vi "eyecat MAX v2_JS-Demo.vi"() -> ()   [LabVIEW 2014]
doc: "This VI is an upgrade from the WIN 1_v4 that implements the ageing subrutine"
uses:
  Buttons/String output.ctl
  <vilib>/Utility/miscctls.llb/LVRowAndColumnTypeDef.ctl
  Buttons/Numeric control.ctl
  Buttons/String input.ctl
  Buttons/Numeric indicator.ctl
  Controls Win/Control 3.ctl
  <vilib>/Platform/TimedLoop/XDataNode/nitl_modes.ctl
  <vilib>/Platform/TimedLoop/XDataNode/timing_clust.ctl
  <vilib>/Platform/TimedLoop/XDataNode/wakeup.ctl
  <vilib>/Utility/file.llb/Read From Spreadsheet File (DBL).vi
  <vilib>/Utility/file.llb/Write To Spreadsheet File (string).vi
  <vilib>/Utility/file.llb/Read From Spreadsheet File (string).vi
  <vilib>/regexp/Match Regular Expression.xnode
  <vilib>/Platform/TimedLoop/XDataNode/XDataNode.xnode
  <vilib>/Platform/TimedLoop/XDataNode/XDNodeRunTimeDep.lvlib
panel:
  in  "System Guide":bool
  in  "Mean(Off)/Interval(On) 5":bool
  in  "System Band":dbl=1.04
  in  "System Sync":i32
  in  "Heat Guide":bool
  in  "Mean(Off)/Interval(On) 4":bool
  in  "Heat Band %":dbl=1.04
  in  "Heat Sync":i32
  in  "Lambda Guide":bool
  in  "Mean(Off)/Interval(On) 3":bool
  in  "Lambda Band %":dbl=1.04
  in  "Lambda Sync":i32
  in  "FlowGuide":bool
  in  "Mean(Off)/Interval(On) 2":bool
  in  "Flow Band %":dbl=1.04
  in  "Flow Sync":i32
  in  "Execute Leak Test Button":bool
  in  "Stop Test Button":bool
  in  "Start Test Button":bool
  in  "Log Test Button":bool
  in  "Boolean":bool
  in  "MKS":bool
  in  "7170":bool
  out "Emissions":dbl[](array[numeric])
  in  "Temperature Sync":i32
  in  "TempGuide":bool
  in  "Temp Band %":dbl=1.04
  in  "Mean(Off)/Interval(On)":bool
  in  "MKS":bool
  out "output cluster":T2
  out "Lambda":dbl[](array[numeric])
  out "MKS HC":dbl
  in  "HC Index":i32
  in  "MFC Number":i32
  out "Open/Closed \nLoop":dbl[](array[numeric])
  out "Air Cyc 2":dbl[](array[numeric])
  in  "Cycle size":i32
  out "MFC Setpoint/Delivery":dynamicdata(graph)
  out "ExtAnDn":bool
  out "ExtAnUp":bool
  out "HC Cyc 2":dbl[](array[numeric])
  out "SO Valve 2":dbl[](array[numeric])
  out "SO Valve 1":dbl[](array[numeric])
  out "Air Bal":dbl[](array[numeric])
  out "HC Bal":dbl[](array[numeric])
  out "Air Cyc 1":dbl[](array[numeric])
  out "HC Cyc 1":dbl[](array[numeric])
  out "File name":string
  out "Log?":bool
  out "Advanced Logging":bool
  out "Connected":bool
  out "MKS 1":i16
  out "MKS 2":i16
  out "Furnace temp 2":dbl
  out "Full system?":bool
  out "Log interval (seconds)":T1
  in  "Flow rate Age":dbl
  in  "Inlet temp Age":dbl
  out "Stopped?":bool
  in  "Stop Cmd":T1
  out "Connected?":bool
  out "Error":dbl
  out "Iteration Duration":i64
  out "Finished Late? [i-1]":bool
  in  "SO2 ppm":dbl
  out "Furnace temp 1":dbl
  out "stop 2":bool
  in  "Enum 1":i16=1
  in  "Acknowledge":bool
  out "Test number":u16
  out "Flag1":bool=TRUE
  out "EditPos Subc":T3
  out "Flag 2":bool=TRUE
  in  "Tab Control":T4(tab)
  in  "Leak Test":bool
  in  "Stop Test":bool
  in  "Log Test Data":bool
  in  "Start":bool
  in  "Adv Settings":bool
  out "Doors Unlocked":bool
  in  "Temperature Limit (°C)":T1=800.0 min=0.0 max=1200.0 step=1.0
  in  "File Name":T5="Test"
  in  "File Path":path=path "C:/DATA LOG"
  out "Fail":bool
  out "Pass":bool
  in  "Select Test Type":T6(radio)
  out "Standby":bool
  out "Doors Open":bool
  out "Extractor Fan On":bool
  out "Test In Progress":bool
  out "Cool Down":bool
  out "System Alarm":bool
  in  "Inlet Temperature (°C)":T1=400.0 min=350.0 max=1000.0 step=1.0
  in  "Inlet LAMBDA Rich":T1=0.9 min=0.85 max=0.96 step=0.001
  in  "Inlet LAMBDA Lean":T1=1.2 min=1.02 max=3.0 step=0.001
  in  "Test Stop temperature (°C)":T1=300.0 min=100.0 max=1000.0 step=1.0
  in  "Test Start Temperature (°C)":T1=125.0 min=0.0 max=500.0 step=1.0
  in  "Furnace Ramp Rate (°C/min)":T1=15.0 min=1.0 max=50.0 step=0.1
  in  "NO:CO Ratio":T1=1.1 min=1.0 max=5.0 step=0.1
  in  "Inlet O2 (%)":T1=0.5 min=0.0 max=14.0 step=0.01
  in  "Inlet LAMBDA":T1=1.0 min=0.6 max=3.0 step=0.001
  out "Space Velocity (h-1)":T7
  out "Vol Flow @ STP (l/min)":T7
  in  "Test Flow Rate(g/s)":T1 min=0.0 max=100.0 step=0.01
  out "Sample Volume (litres)":T7
  in  "Number of Samples":T1=1.0 min=1.0 max=6.0 step=1.0
  in  "Sample Diameter (mm)":T1
  out "CO Theory (%)":T7 format="%#_3g"
  out "CO Theory (%)":T7 format="%#_3g"
  out "HC Theory (%)":T7
  in  "Sample Length (mm)":T1 min=0.0 step=0.5
  in  "NO ppm SW":dbl=500.0 caption="NO (ppm)" min=0.0 max=500.0 step=1.0
  in  "NO ppm Loff":T1 caption="NO ppm"
  in  "Delete sCycle":bool
  in  "Load sCycle":bool
  in  "Save sCycle":bool
  in  "Clear subcycle":bool
  in  "Clear Cycle Pattern":bool
  in  "Save Cycle":bool
  in  "Load Cycle":bool
  in  "Delete Cycle":bool
  out "Test Compiled":bool
  in  "Compile Test Button":bool
  in  "Sub-Cycle List":i32(listbox)=1
  in  "Cycle List":i32(listbox)=2
  out "Total Test Duration (hrs)":T8
  in  "Ageing Gas":enum32{"Radio Selection 1", "Radio Selection 2"}(radio)
  in  "Sub-Cycle Pattern":string[][](table) caption="Subcycle pattern"
  in  "Total Number of Cycles":T1=1.0 min=1.0 max=10000.0 step=1.0
  in  "Cycle Pattern":string[][](table)
  in  "Sub-Cycle Name":T5
  in  "Cycle Name":T5
  out "Heat Exchanger Temperatures (°C)":dynamicdata(graph)
  out "Flow Rate (g/s)":dynamicdata(graph)
  out "Sample Temperatures (°C)":dynamicdata(graph)
  out "System Temperatures (°C)":dynamicdata(graph)
  out "HC Concentration (ppm)":dynamicdata(graph)
  out "Lambda":dynamicdata(graph)
  out "M584L Upstream & Downstream":dynamicdata(graph)
  out "NO Concentration (ppm)":dynamicdata(graph)
  in  "Purge System":bool
  in  "Alarm ack":bool
  in  "Clear log":bool
  out "Table":string[][](table)
  out "Soft Alarm":bool
  out "Hard Alarm":bool
  # "0 HC Cyc 1\n1 Air Cyc 1\n2 Air Bal\n3 HC Bal\n4 Air Cyc 2\n5 HC Cyc 2"
  # "1% = 0.01"
  # "Test Type"
  # "Test Commands"
  # "System Indicators"
  # "Leak Test"
  # "Catalyst Specification"
  # "Lightoff Settings"
  # "Furnace Lightoff Settings"
  # "Sweep Settings"
  # "CO/HC Lightoff Settings"
  # "0.96 < lambda < 0.85"
  # "1.02< lambda < 1.6"
  # "350 < Tinlet < 1000"
  # "NO Lightoff Settings"
  # "Flow Specification"
  # "Cycle Compiled"
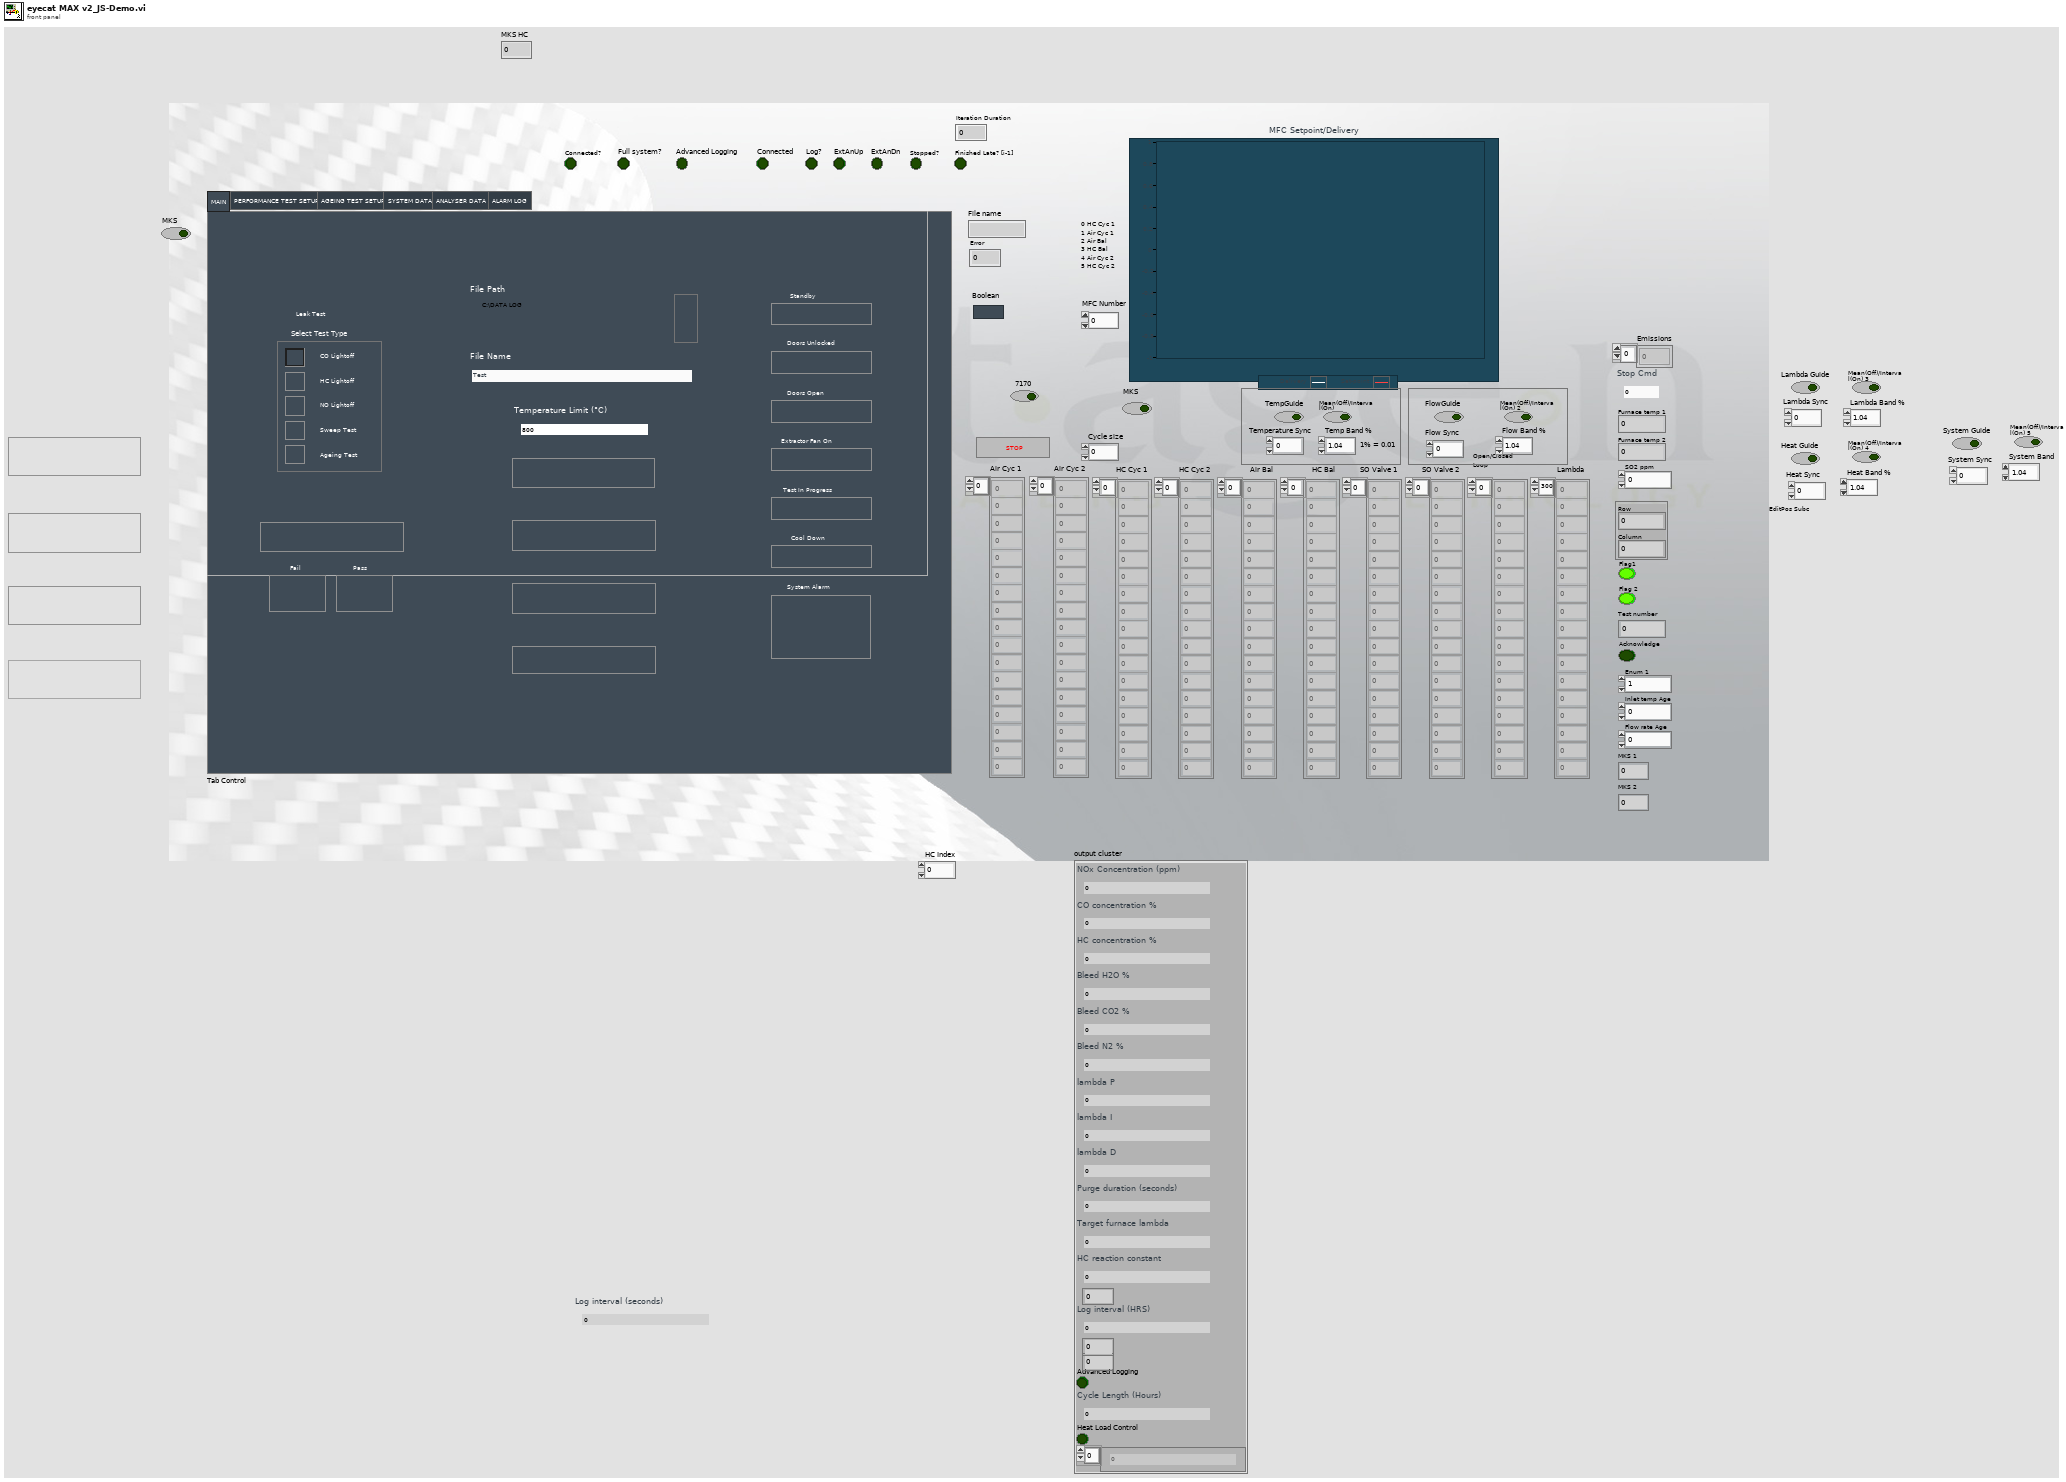
[diagram p1: front panel]
types:
  T1 = typedef "Numeric control.ctl" = dbl
  T2 = cluster{"NOx Concentration (ppm)":T1, "CO concentration %":T1, "HC concentration %":T1, "Bleed H2O %":T1, "Bleed CO2 %":T1, "Bleed N2 %":T1, "lambda P":T1, "lambda I":T1, "lambda D":T1, "Purge duration (seconds)":T1, "Target furnace lambda":T1, "HC reaction constant":T1, i16, "Log interval (HRS)":T1, i16, i16, "Advanced Logging":bool, "Cycle Length (Hours)":T1, "Heat Load Control":bool, T1[]}
  T3 = typedef "LVRowAndColumnTypeDef.ctl" = cluster{"Row":i32, "Column":i32}
  T4 = enum32{"MAIN", "PERFORMANCE TEST SETUP", "AGEING TEST SETUP", "SYSTEM DATA", "ANALYSER DATA", "ALARM LOG"}
  T5 = typedef "String input.ctl" = string
  T6 = enum32{"CO Lightoff", "HC Lightoff", "NO Lightoff", "Sweep Test", "Ageing Test"}
  T7 = typedef "Numeric indicator.ctl" = dbl
  T8 = typedef "String output.ctl" = string
  T9 = typedef "XDNodeRunTimeDep.lvlib/nitl_modes.ctl" = enum32{"No Change", "Process missed periods, maintain original phase", "Discard missed periods, maintain original phase", "Process missed periods, ignore original phase", "Discard missed periods, ignore original phase"}
  T10 = typedef "Control 3.ctl" = enum16{"main", "start test", "save subc", "load subc", "delete subc", "clear table 1", "update list 1", "save cycle", "load cycle", "delete cycle", "clear table 2", "update list 2", "calc HC CO", "Total time calc", "update Cycle pattern ", "load cycle name", "convert to num", "load test array", "check scycle name", "check cycle name", "Multigas connect", "Multigas disconnect"}
  T11 = enum8{"Enabled", "Disabled", "Disabled and Grayed Out"}
  T12 = typedef "XDNodeRunTimeDep.lvlib/timing_clust.ctl" = cluster{"Expected End [f-1]":u64, "Actual End [f-1]":u64, "Finished Late? [f-1]":bool, "Expected End [i-1]":u64, "Actual End [i-1]":u64, "Finished Late? [i-1]":bool, "Expected Start [i]":u64, "Actual Start [i]":u64, "Expected Start [f]":u64, "Actual Start [f]":u64, "Source Name":string, "Structure Name":string, "Period":i64, "Deadline":i64, "Offset":i64, "Start":i64, "Priority":i32, "Timeout":i32, "Mode":T9, "Wakeup Reason":T13, "Error":errorcluster, "Source Type":string, "Secondary Source Type":string, "Global End Time":u64, "Global Start Time":u64, "Frame Duration":u64, "Iteration Duration":u64, "Assigned CPU":i32, "I/O Scan Engine Mode":u32}
  T13 = typedef "XDNodeRunTimeDep.lvlib/wakeup.ctl" = enum32{"Normal", "Aborted", "Asynchronous wakeup", "Timing source error", "Timed loop error", "Timeout"}
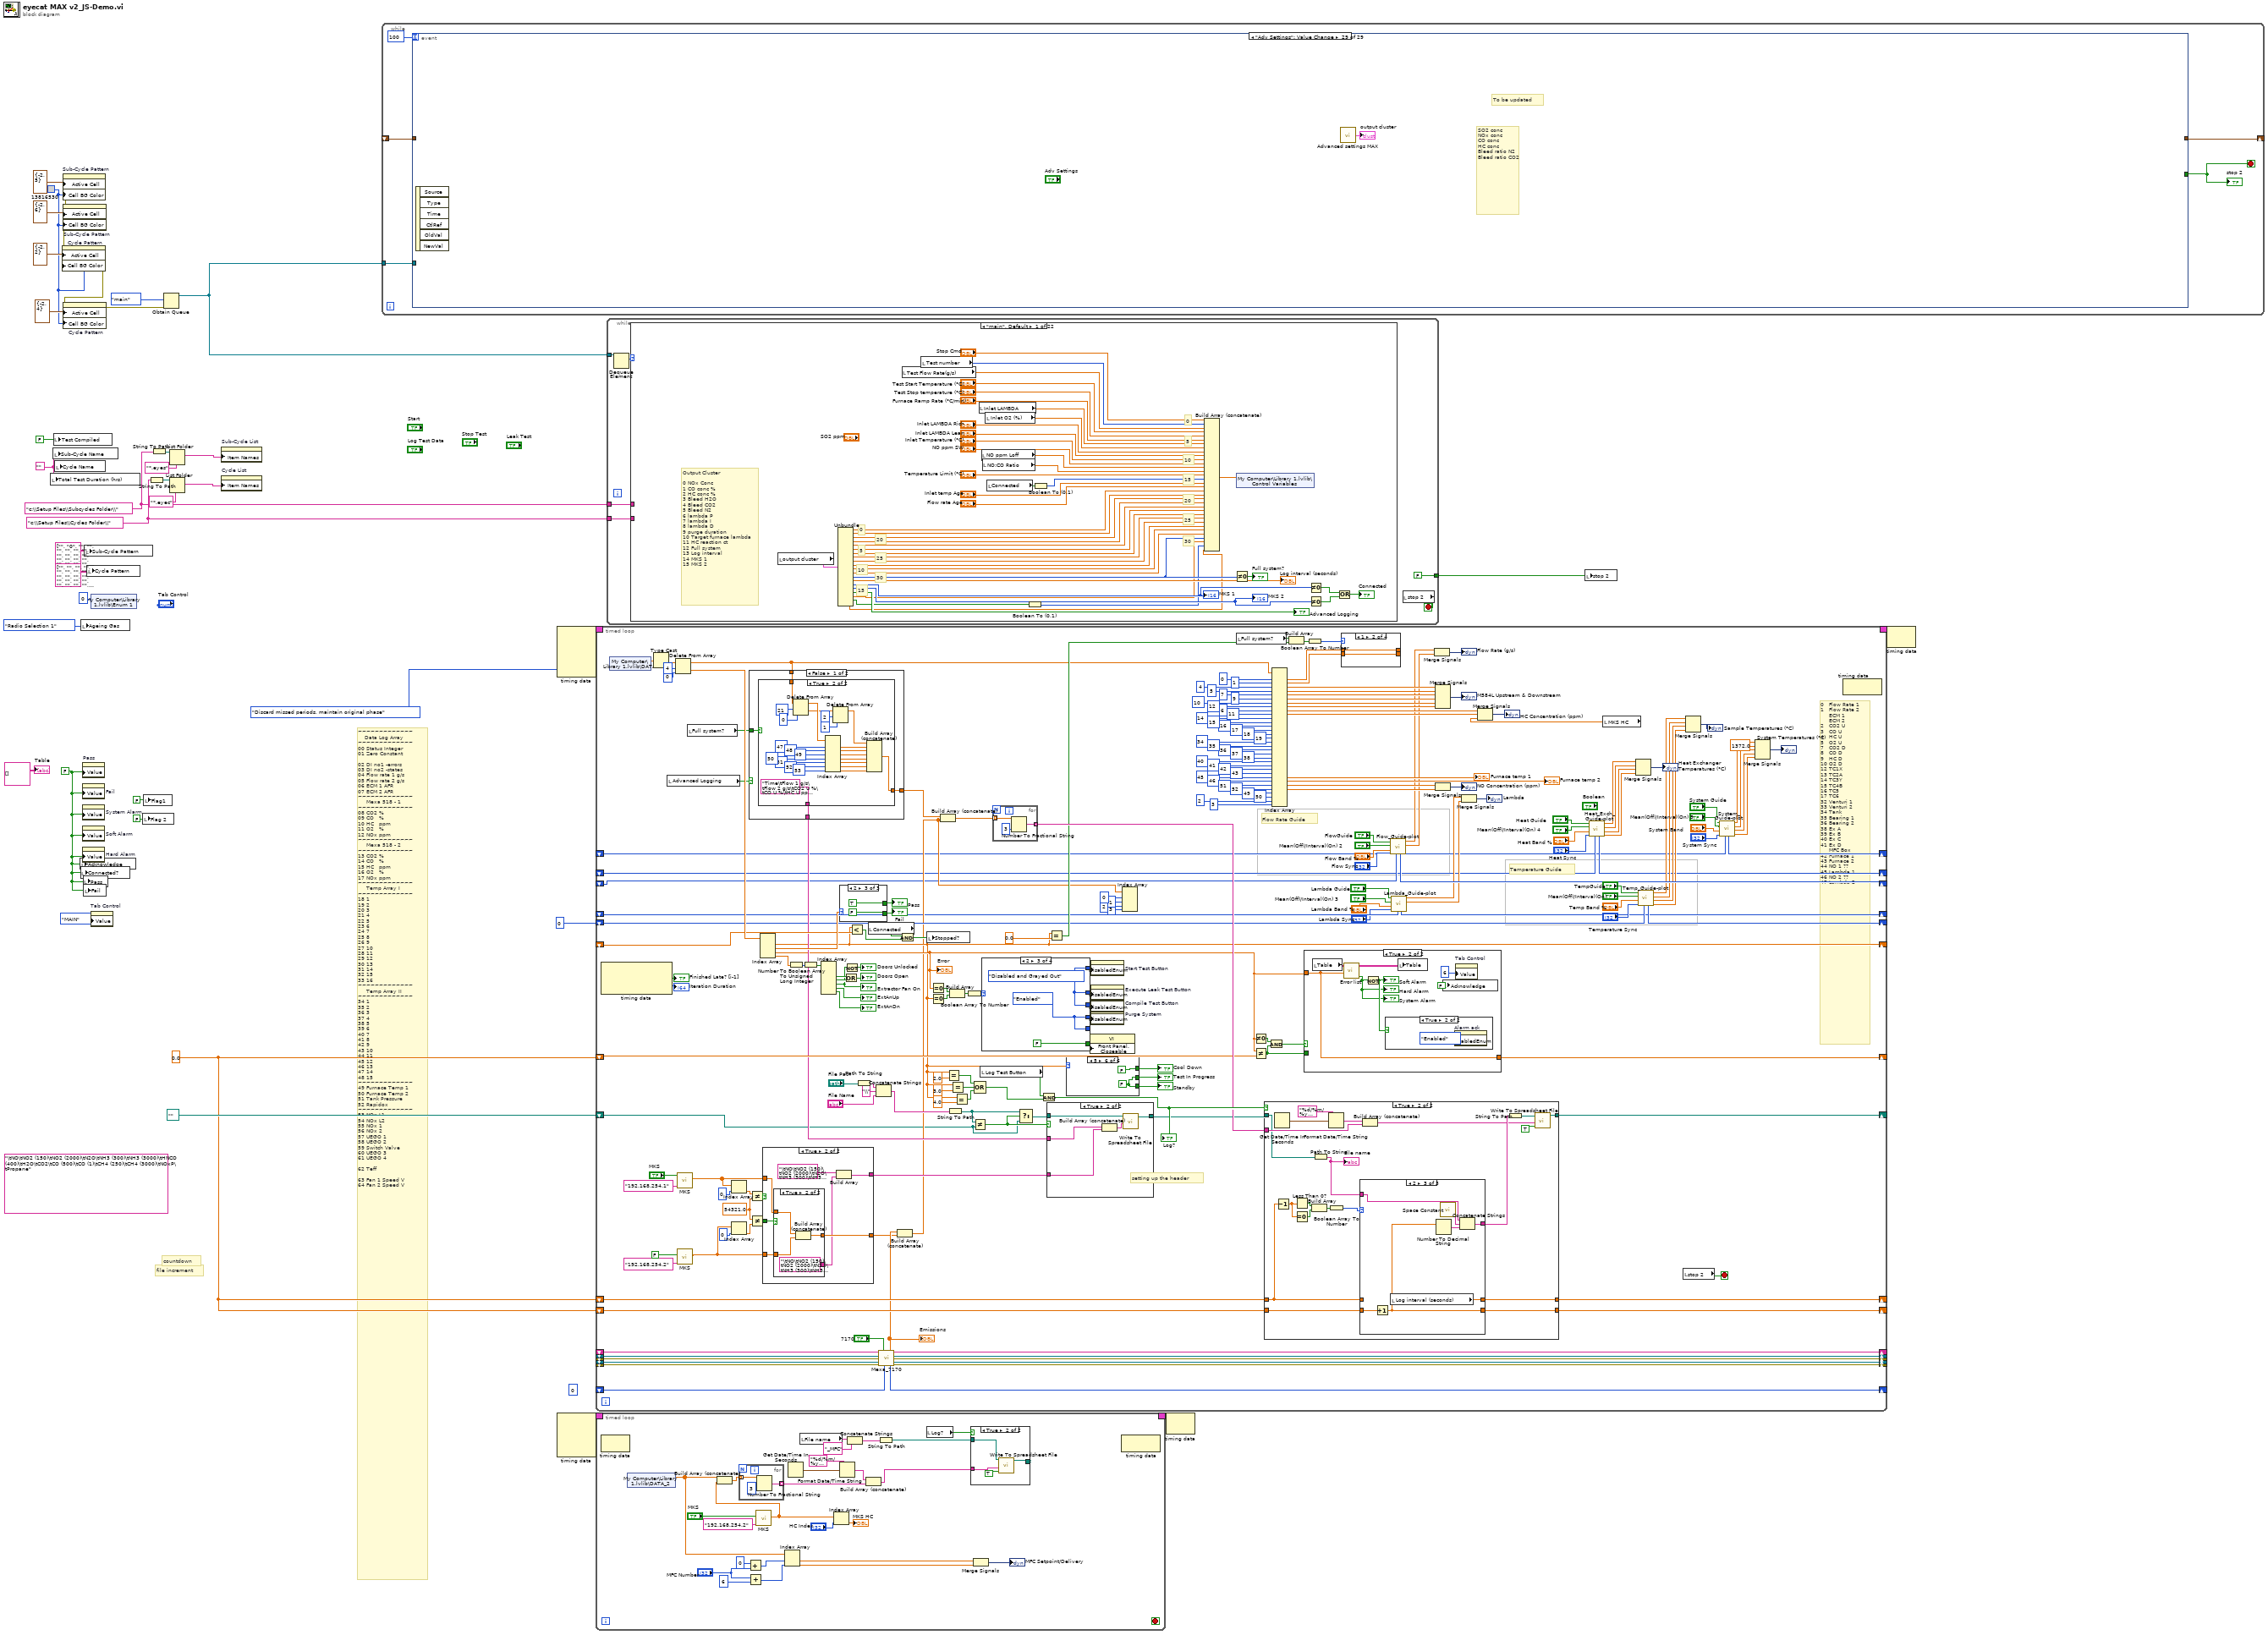
[diagram p0: block diagram]
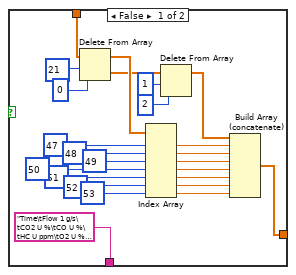
[diagram p3: hidden frame]
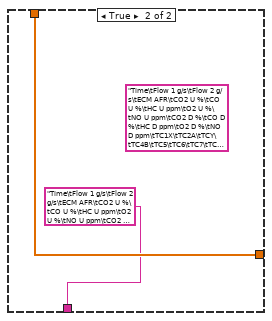
[diagram p4: hidden frame]
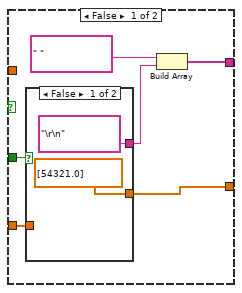
[diagram p5: hidden frame]
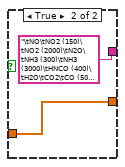
[diagram p6: hidden frame]
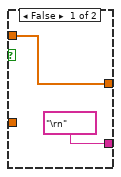
[diagram p7: hidden frame]
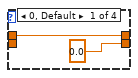
[diagram p8: hidden frame]
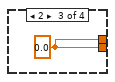
[diagram p9: hidden frame]
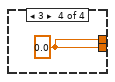
[diagram p10: hidden frame]
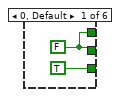
[diagram p11: hidden frame]
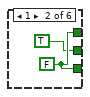
[diagram p12: hidden frame]
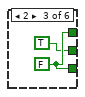
[diagram p13: hidden frame]
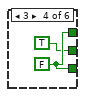
[diagram p14: hidden frame]
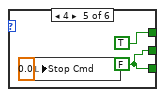
[diagram p15: hidden frame]
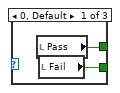
[diagram p16: hidden frame]
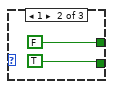
[diagram p17: hidden frame]
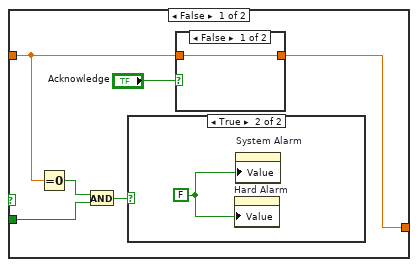
[diagram p18: hidden frame]
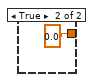
[diagram p19: hidden frame]
diagram:
  (unwired) 0 ("index")
  (unwired) "\tNO\tNO2 (150)\tNO2 (2000)\tN2O\tNH3 (300)\tNH3 (3000)\tHNCO (400)\tH2O\tCO2\tCO (500)\tCO (1)\tCH4 (250)\tCH4 (3000)\tNOxP\tPropane" ("Heading string 2")
  w5 = FALSE
  w4 = 0.0 ("y")
  w21 = ""
  w24 = "c:\\Setup Files\\Cycles Folder\\"
  w30 = u32 13816530
  w22 = "c:\\Setup Files\\Subcycles Folder\\"
  # "~~~~~~~~~~~~~\n    Data Log Array\n~~~~~~~~~~~~~\n00 Status Integer\n01 Zero Constant\n\n02 DI no1 -errors\n03 DI no2 -states\n04 Flow rate 1 g/s\n05 Flow rate 2 g/s\n06 ECM 1 AFR\n07 ECM 2 AFR\n~~~~~~~~~~~~~\n     Mexa 518 - 1\n~~~~~~~~~~~~~\n08 CO2 %\n09 CO   %\n10 HC   ppm\n11 O2   %\n12 NOx ppm\n~~~~~~~~~~~~~\n     Mexa 518 - 2\n~~~~~~~~~~~~~\n13 CO2 %\n14 CO   %\n15 HC   ppm\n16 O2   %\n17 NOx ppm\n~~~~~~~~~~~~~\n     Temp Array I\n~~~~~~~~~~~~~\n18 1\n19 2 \n20 3\n21 4\n22 5\n23 6\n24 7\n25 8\n26 9\n27 10\n28 11\n29 12\n30 13\n31 14\n32 15\n33 16\n~~~~~~~~~~~~~\n     Temp Array II\n~~~~~~~~~~~~~\n34 1\n35 2\n36 3\n37 4\n38 5\n39 6\n40 7\n41 8\n42 9\n43 10\n44 11\n45 12\n46 13\n47 14\n48 15\n~~~~~~~~~~~~~\n49 Furnace Temp 1\n50 Furnace Temp 2\n51 Tank Pressure\n52 Rapidox\n~~~~~~~~~~~~~\n53 NOx L1\n54 NOx L2\n55 NOx 1\n56 NOx 2\n57 UEGO 1\n58 UEGO 2\n59 Switch Valve\n60 UEGO 3\n61 UEGO 4\n\n62 Teff\n\n63 Fan 1 Speed V\n64 Fan 2 Speed V"
  # "file increment"
  # "countdown"
  n1 = local write "Total Test Duration (hrs)"(w21) -> ()
  n2 = local write "Sub-Cycle Name"(w21) -> ()
  n3 = local write "Test Compiled"(FALSE ("Cycle Compiled")) -> ()
  n4 = local write "Cycle Name"(w21) -> ()
  n5 = property on="Sub-Cycle Pattern" class="Tbl (strict)"("Active Cell"=T3 {"Row"=-2, "Column"=5} ("Active Cell:Active Cell"), "Cell BG Color"=w30) -> (error out=w35:errorcluster)  [unwired: 2 in, 1 out]
  n6 = property on="Sub-Cycle Pattern" class="Tbl (strict)"(error in=w35, "Active Cell"=T3 {"Row"=-2, "Column"=6} ("Active Cell:Active Cell"), "Cell BG Color"=w30) -> (error out=w34:errorcluster)  [unwired: 1 in, 1 out]
  n7 = property on="Cycle Pattern" class="Tbl (strict)"(error in=w34, "Active Cell"=T3 {"Row"=-2, "Column"=2} ("Active Cell:Active Cell"), "Cell BG Color"=w30) -> (error out=w32:errorcluster)  [unwired: 1 in, 1 out]
  n8 = property on="Cycle Pattern" class="Tbl (strict)"(error in=w32, "Active Cell"=T3 {"Row"=-2, "Column"=4} ("Active Cell:Active Cell"), "Cell BG Color"=w30) -> (error out=w29:errorcluster)  [unwired: 1 in, 1 out]
  n9 = local write "Acknowledge"(w5) -> ()
  n10 = local write "Connected?"(w5) -> ()
  n11 = local write "Ageing Gas"(enum32{"Radio Selection 1", "Radio Selection 2"}."Radio Selection 1" ("Ageing Gas")) -> ()
  n12 = property on="Pass" class="Bool (strict)"("Value"=w5) -> ()  [unwired: 2 in, 2 out]
  n13 = property on="Fail" class="Bool (strict)"("Value"=w5) -> ()  [unwired: 2 in, 2 out]
  n14 = property on="System Alarm" class="Bool (strict)"("Value"=w5) -> ()  [unwired: 2 in, 2 out]
  n15 = property on="Soft Alarm" class="Bool (strict)"("Value"=w5) -> ()  [unwired: 2 in, 2 out]
  n16 = property on="Hard Alarm" class="Bool (strict)"("Value"=w5) -> ()  [unwired: 2 in, 2 out]
  n17 = local write "Pass"(w5) -> ()
  n18 = local write "Fail"(w5) -> ()
  n19 = local write "Sub-Cycle Pattern"(string[][] [["", "0", "", "", "", "", "", "", "", "", "", "", ""], ["", "", "", "", "", "", "", "", "", "", "", "", ""], ["", "", "", "", "", "", "", "", "", "", "", "", ""], ["", "", "", "", "", "", "", "", "", "", "", "", ""], ["", "", "", "", "", "", "", "", "", "", "", "", ""], ["", "", "", "", "", "", "", "", "", "", "", "", ""], ["", "", "", "", "", "", "", "", "", "", "", "", ""], ["", "", "", "", "", "", "", "", "", "", "", "", ""], ["", "", "", "", "", "", "", "", "", "", "", "", ""], ["", "", "", "", "", "", "", "", "", "", "", "", ""], ["", "", "", "", "", "", "", "", "", "", "", "", ""], ["", "", "", "", "", "", "", "", "", "", "", "", ""], ["", "", "", "", "", "", "", "", "", "", "", "", ""], ["", "", "", "", "", "", "", "", "", "", "", "", ""], ["", "", "", "", "", "", "", "", "", "", "", "", ""], ["", "", "", "", "", "", "", "", "", "", "", "", ""], ["", "", "", "", "", "", "", "", "", "", "", "", ""], ["", "", "", "", "", "", "", "", "", "", "", "", ""], ["", "", "", "", "", "", "", "", "", "", "", "", ""], ["", "", "", "", "", "", "", "", "", "", "", "", ""], ["", "", "", "", "", "", "", "", "", "", "", "", ""], ["", "", "", "", "", "", "", "", "", "", "", "", ""], ["", "", "", "", "", "", "", "", "", "", "", "", ""], ["", "", "", "", "", "", "", "", "", "", "", "", ""], ["", "", "", "", "", "", "", "", "", "", "", "", ""], ["", "", "", "", "", "", "", "", "", "", "", "", ""], ["", "", "", "", "", "", "", "", "", "", "", "", ""], ["", "", "", "", "", "", "", "", "", "", "", "", ""], ["", "", "", "", "", "", "", "", "", "", "", "", ""], ["", "", "", "", "", "", "", "", "", "", "", "", ""], ["", "", "", "", "", "", "", "", "", "", "", "", ""]]) -> ()
  n20 = local write "Cycle Pattern"(string[][] [["", "", "", "", ""], ["", "", "", "", ""], ["", "", "", "", ""], ["", "", "", "", ""], ["", "", "", "", ""], ["", "", "", "", ""], ["", "", "", "", ""], ["", "", "", "", ""], ["", "", "", "", ""], ["", "", "", "", ""], ["", "", "", "", ""], ["", "", "", "", ""], ["", "", "", "", ""], ["", "", "", "", ""], ["", "", "", "", ""], ["", "", "", "", ""], ["", "", "", "", ""], ["", "", "", "", ""], ["", "", "", "", ""], ["", "", "", "", ""], ["", "", "", "", ""], ["", "", "", "", ""], ["", "", "", "", ""], ["", "", "", "", ""], ["", "", "", "", ""], ["", "", "", "", ""], ["", "", "", "", ""], ["", "", "", "", ""], ["", "", "", "", ""], ["", "", "", "", ""], ["", "", "", "", ""]]) -> ()
  n21 = shared-variable "My Computer\\Library 1.lvlib\\Enum 1"(u16 0 ("Enum 1")) -> ()  [unwired: 1 in, 1 out]
  n22 = property on="Tab Control" class="TabCtl (strict)"("Value"=T4."MAIN" ("Tab Control")) -> ()  [unwired: 2 in, 2 out]
  n23 = local write "Flag 2"(FALSE) -> ()
  n24 = local write "Flag1"(FALSE) -> ()
  n25 = String To Path(string=w24) -> (path=w25:path)
  n26 = String To Path(string=w22) -> (path=w27:path)
  n27 = Obtain Queue(element data type=Control_3."main" ("Enum"), error in (no error)=w29) -> (queue out=w38:refnum<queue>)  [unwired: 3 in, 2 out]
  n28 = List Folder(path=w25, pattern="*.eyec") -> (filenames=w26:string[])  [unwired: 2 in, 3 out]
  n29 = List Folder(path=w27, pattern="*.eyes") -> (filenames=w28:string[])  [unwired: 2 in, 3 out]
  n30 = property on="Sub-Cycle List" class="LstBox (strict)"("Item Names"=w28) -> ()  [unwired: 2 in, 2 out]
  n31 = property on="Cycle List" class="LstBox (strict)"("Item Names"=w26) -> ()  [unwired: 2 in, 2 out]
  n32 = while {
    tunnel: w38 -> [w44]
    shift-right: [w42] -> _
    shift-left: _ -> [w41]
    stop <- w40 stop-if-true
    n33 = event shown="[28] \"Adv Settings\": Value Change" {
      selector: _ -> [_ _ _ _ _ _ _ _ _ _ _ _ _ _ _ _ _ _ _ _ _ _ _ _ _ _ _ _ _]
      dyn-events: _ -> [_ _ _ _ _ _ _ _ _ _ _ _ _ _ _ _ _ _ _ _ _ _ _ _ _ _ _ _ _]
      timeout: 100 -> [_ _ _ _ _ _ _ _ _ _ _ _ _ _ _ _ _ _ _ _ _ _ _ _ _ _ _ _ _]
      tunnel: w44 -> [w47 w49 _ w58 w66 w73 w80 w91 w95 w106 w111 w114 w119 w141 w149 w150 _ _ _ _ w194 w210 _ w287 w305 _ w319 _ _]
      tunnel: [w45 w48 _ w59 w65 w72 w79 w90 w93 w101 w108 w113 w117 w138 _ _ _ _ _ _ _ _ _ _ _ _ _ _ _] -> w42
      tunnel: w41 -> [w45 w48 _ w59 w65 w72 w78 w90 w93 w101 w108 w113 w117 w138 _ _ _ _ _ _ _ _ _ _ _ _ _ _ _]
      tunnel: [_ _ w51 _ _ _ _ _ _ _ _ _ _ _ _ _ _ _ _ _ _ _ _ _ _ _ _ _ _] -> w40
      event Timeout {
        n34 = event-data() -> ()  [unwired: 1 in, 2 out]
        n35 = Enqueue Element(queue=w47, element=Control_3."main" ("Enum")) -> ()  [unwired: 2 in, 3 out]
      }
      event "Clear subcycle": Value Change {
        n36 = event-data() -> ()  [unwired: 1 in, 5 out]
        n37 = Enqueue Element(queue=w49, element=Control_3."clear table 1" ("Enum")) -> ()  [unwired: 2 in, 3 out]
      }
      event Panel Close? {
        n38 = event-data() -> ()  [unwired: 1 in, 3 out]
        n39 = Two Button Dialog(message="This command will close Eyecat!\nDo you wish to continue?", 1:"No" ("F button name (\"Cancel\")"), 2:"Yes" ("T button name (\"OK\")")) -> (T button?=w51:bool)
        n40 = Not(x=w51) -> (.not. x?=w52:bool)
        n41 = event-data("Discard?"=w52) -> ()  [unwired: 1 in, 1 out]
      }
      event "Save sCycle": Value Change {
        n42 = event-data() -> ()  [unwired: 1 in, 5 out]
        n43 = local read "Sub-Cycle Pattern"() -> (w56:string[][])
        n44 = call "Time column check.vi"("Array"=w56) -> ("Mistake?"=w57:bool)  [unwired: 10 in]
        n45 = case shown="False" w57 {
          tunnel: w58 -> [w60 _]
          frame False {
            n46 = Enqueue Element(queue=w60, element=Control_3."save subc") -> (queue out=w62:refnum<queue>)  [unwired: 2 in, 2 out]
            n47 = Enqueue Element(queue=w62, element=Control_3."update list 1") -> ()  [unwired: 2 in, 3 out]
          }
          frame True {
            n48 = One Button Dialog(message="The time sequence is incorrect!\nReview and save again!") -> ()  [unwired: 1 in, 1 out]
          }
        }
      }
      event "Load sCycle": Value Change {
        n49 = event-data() -> ()  [unwired: 1 in, 5 out]
        n50 = Enqueue Element(queue=w66, element=Control_3."load subc") -> ()  [unwired: 2 in, 3 out]
      }
      event "Delete sCycle": Value Change {
        n51 = event-data() -> ()  [unwired: 1 in, 5 out]
        n52 = Enqueue Element(queue=w73, element=Control_3."delete subc") -> (queue out=w75:refnum<queue>)  [unwired: 2 in, 2 out]
        n53 = Enqueue Element(queue=w75, element=Control_3."update list 1") -> (queue out=w71:refnum<queue>)  [unwired: 2 in, 2 out]
        n54 = Enqueue Element(queue=w71, element=Control_3."update Cycle pattern ") -> (queue out=w68:refnum<queue>)  [unwired: 2 in, 2 out]
        n55 = Enqueue Element(queue=w68, element=Control_3."Total time calc") -> ()  [unwired: 2 in, 3 out]
      }
      event "Sub-Cycle Pattern": Mouse Down; "Sub-Cycle Pattern": Value Change {
        n56 = event-data() -> ()  [unwired: 1 in, 3 out]
        n57 = property on="Sub-Cycle Pattern" class="Tbl (strict)"() -> ("EditPos"=w79:T3)  [unwired: 2 in, 2 out]
        n58 = Unbundle By Name(w79) -> ("Row"=w81:i32)  [unwired: 1 out]
        n59 = Less?(x=w81, y=30) -> (x < y?=w83:bool)
        n60 = case shown="True" w83 {
          tunnel: w80 -> [_ w88]
          frame False {
            n61 = One Button Dialog(message="This table is limited to 30 entries!") -> ()  [unwired: 1 in, 1 out]
          }
          frame True {
            n62 = Enqueue Element(queue=w88, element=Control_3."convert to num") -> (queue out=w87:refnum<queue>)  [unwired: 2 in, 2 out]
            n63 = Enqueue Element(queue=w87, element=Control_3."calc HC CO") -> ()  [unwired: 2 in, 3 out]
          }
        }
        "EditPos Subc" <- w78
        "Flag1" <- TRUE
      }
      event "Clear Cycle Pattern": Value Change {
        n64 = event-data() -> ()  [unwired: 1 in, 5 out]
        n65 = Enqueue Element(queue=w91, element=Control_3."clear table 2" ("Enum")) -> ()  [unwired: 2 in, 3 out]
        n66 = local write "Test Compiled"(FALSE ("Test Compiled")) -> ()
      }
      event "Save Cycle": Value Change {
        n67 = event-data() -> ()  [unwired: 1 in, 5 out]
        n68 = Enqueue Element(queue=w95, element=Control_3."update Cycle pattern ") -> (queue out=w94:refnum<queue>)  [unwired: 2 in, 2 out]
        n69 = Enqueue Element(queue=w94, element=Control_3."save cycle") -> (queue out=w98:refnum<queue>)  [unwired: 2 in, 2 out]
        n70 = Enqueue Element(queue=w98, element=Control_3."update list 2") -> ()  [unwired: 2 in, 3 out]
      }
      event "Load Cycle": Value Change {
        n71 = event-data() -> ()  [unwired: 1 in, 5 out]
        n72 = Enqueue Element(queue=w106, element=Control_3."load cycle") -> (queue out=w104:refnum<queue>)  [unwired: 2 in, 2 out]
        n73 = Enqueue Element(queue=w104, element=Control_3."update Cycle pattern ") -> (queue out=w103:refnum<queue>)  [unwired: 2 in, 2 out]
        n74 = local write "Test Compiled"(FALSE ("Test Compiled")) -> ()
        n75 = Enqueue Element(queue=w103, element=Control_3."Total time calc") -> ()  [unwired: 2 in, 3 out]
      }
      event "Delete Cycle": Value Change {
        n76 = event-data() -> ()  [unwired: 1 in, 5 out]
        n77 = Enqueue Element(queue=w111, element=Control_3."delete cycle") -> (queue out=w110:refnum<queue>)  [unwired: 2 in, 2 out]
        n78 = Enqueue Element(queue=w110, element=Control_3."update list 2") -> ()  [unwired: 2 in, 3 out]
      }
      event Value Change {
        n79 = event-data() -> ()  [unwired: 1 in, 5 out]
        n80 = Enqueue Element(queue=w114, element=Control_3."Total time calc") -> ()  [unwired: 2 in, 3 out]
      }
      event "Cycle Pattern": Mouse Up; "Cycle Pattern": Value Change {
        n81 = event-data() -> ()  [unwired: 1 in, 3 out]
        n82 = property on="Cycle Pattern" class="Tbl (strict)"() -> ("EditPos"=w121:T3)  [unwired: 2 in, 2 out]
        n83 = Unbundle By Name(w121) -> ("Row"=w118:i32, "Column"=w123:i32)
        n84 = Less?(x=w118, y=30) -> (x < y?=w122:bool)
        n85 = case shown="True" w122 {
          tunnel: w123 -> [_ w125]
          tunnel: w119 -> [_ w128]
          frame False {
            n86 = One Button Dialog(message="This table is limited to 30 entries!") -> ()  [unwired: 1 in, 1 out]
          }
          frame True {
            n87 = Equal?(x=w125, y=1) -> (x = y?=w129:bool)
            n88 = case shown="True" w129 {
              tunnel: w128 -> [w132 w135]
              tunnel: [w131 w134] -> w127
              frame False {
                n89 = Enqueue Element(queue=w132, element=Control_3."update Cycle pattern ") -> (queue out=w131:refnum<queue>)  [unwired: 2 in, 2 out]
              }
              frame True {
                n90 = Enqueue Element(queue=w135, element=Control_3."load cycle name") -> (queue out=w134:refnum<queue>)  [unwired: 2 in, 2 out]
              }
            }
            n91 = Enqueue Element(queue=w127, element=Control_3."Total time calc") -> ()  [unwired: 2 in, 3 out]
          }
        }
        "Flag 2" <- TRUE
      }
      event "Compile Test Button": Value Change {
        n92 = event-data() -> ()  [unwired: 1 in, 5 out]
        n93 = local read "Flag 2"() -> (w137:bool)
        n94 = case shown="True" w137 {
          tunnel: w141 -> [w142 w146]
          tunnel: [w142 w143] -> w139
          frame False {
          }
          frame True {
            n95 = Enqueue Element(queue=w146, element=Control_3."save cycle") -> (queue out=w144:refnum<queue>)  [unwired: 2 in, 2 out]
            n96 = Enqueue Element(queue=w144, element=Control_3."update list 2") -> (queue out=w143:refnum<queue>)  [unwired: 2 in, 2 out]
          }
        }
        n97 = Enqueue Element(queue=w139, element=Control_3."load test array") -> ()  [unwired: 2 in, 3 out]
      }
      event Value Change {
        n98 = event-data() -> ()  [unwired: 1 in, 5 out]
        n99 = Enqueue Element(queue=w149, element=Control_3."check scycle name") -> ()  [unwired: 2 in, 3 out]
      }
      event Value Change {
        n100 = event-data() -> ()  [unwired: 1 in, 5 out]
        n101 = Enqueue Element(queue=w150, element=Control_3."check cycle name") -> ()  [unwired: 2 in, 3 out]
      }
      event Value Change {
        n102 = event-data() -> ()  [unwired: 1 in, 5 out]
        n103 = Square(x="Sample Diameter (mm)") -> (x^2=w159:T1)
        n104 = Compound Arithmetic op=MULTIPLY(w159, "Sample Length (mm)", "Number of Samples", 3.141592653589793) -> (w158:T1)
        n105 = Divide(x=w158, y=4000000.0) -> (x/y=→"Sample Volume (litres)":T1)
      }
      event Value Change {
        # "O2Eq"
        n106 = event-data() -> ()  [unwired: 1 in, 5 out]
        n107 = local write "Inlet LAMBDA"("Inlet LAMBDA") -> ()
        n108 = local write "Inlet O2 (%)"("Inlet O2 (%)") -> ()
        n109 = Decrement(x="Inlet LAMBDA") -> (x-1=w174:T1)
        n110 = Multiply(x=4.76, y="Inlet LAMBDA") -> (x*y=w170:T1)
        n111 = Multiply(x=w174, y=100.0) -> (x*y=w172:T1)
        n112 = Add(x=0.33, y=w170) -> (x+y=w168:T1)
        n113 = Divide(x=w172, y=w168) -> (x/y=w167:T1)
        n114 = Subtract(x="Inlet O2 (%)", y=w167) -> (x-y=w165:T1)
        n115 = Multiply(x=w165, y=2.0) -> (x*y=→"CO Theory (%)":T1)
        n116 = Divide(x=w165, y=4.5) -> (x/y=→"HC Theory (%)":T1)
      }
      event Value Change {
        n117 = event-data() -> ()  [unwired: 1 in, 5 out]
        n118 = local write "NO ppm Loff"("NO ppm Loff") -> ()
        n119 = local write "NO:CO Ratio"("NO:CO Ratio") -> ()
        n120 = Divide(x="NO ppm Loff", y=T1 10000.0) -> (x/y=w177:T1)
        n121 = Multiply(x="NO:CO Ratio", y=w177) -> (x*y=→"CO Theory (%)":T1)
      }
      event Value Change {
        n122 = event-data() -> ()  [unwired: 1 in, 5 out]
        n123 = local read "Sample Volume (litres)"() -> (w182:T7)
        n124 = Equal?(x=w182, y=0.0) -> (x = y?=w181:bool)
        n125 = case shown="False" w181 {
          tunnel: w182 -> [w187 _]
          tunnel: "Test Flow Rate(g/s)" -> [w184 _]
          frame False {
            w189 = 60.0 ("y")
            n126 = Multiply(x=w184, y=w189) -> (x*y=w191:T1)
            n127 = Divide(x=w191, y=1.2) -> (x/y=w186:T1)
            "Vol Flow @ STP (l/min)" <- w186
            n128 = Multiply(x=w186, y=w189) -> (x*y=w188:T1)
            n129 = Divide(x=w188, y=w187) -> (x/y=→"Space Velocity (h-1)":T1)
          }
          frame True {
            n130 = One Button Dialog(message="Review sample specification first!") -> ()  [unwired: 1 in, 1 out]
          }
        }
      }
      event "Execute Leak Test Button": Value Change {
        n131 = event-data() -> ()  [unwired: 1 in, 5 out]
        n132 = flat-sequence {
          tunnel: w194 -> [w197]
          tunnel: [w197] -> w193
          tunnel: w193 -> [w200]
          frame #0 {
            n133 = local write "Test number"(u16 5) -> ()
            n134 = local write "Enum 1"(u16 3 ("Test number")) -> ()
          }
          frame #1 {
            n135 = Enqueue Element(queue=w200, element=Control_3."main" ("Enum")) -> (queue out=w198:refnum<queue>)  [unwired: 2 in, 2 out]
            n136 = Enqueue Element(queue=w198, element=Control_3."start test" ("Enum")) -> ()  [unwired: 2 in, 3 out]
          }
        }
      }
      event "Start Test Button": Value Change {
        n137 = event-data() -> ()  [unwired: 1 in, 5 out]
        n138 = property on="Log Test Button" class="Bool (strict)"() -> ("Value"=w209:bool)  [unwired: 2 in, 2 out]
        n139 = Boolean To (0,1)(Boolean=w209) -> (0, 1=w208:i16)
        n140 = Equal To 0?(x=w208) -> (x = 0?=w207:bool)
        n141 = case shown="True" w207 {
          tunnel: [TRUE ("T button?") w264] -> w202
          frame False {
          }
          frame True {
            # "Log Data Check"
            n142 = Two Button Dialog(message="You are not currently logging data!\nDo you wish to continue?", 1:"No" ("T button name (\"OK\")"), 2:"Yes" ("T button name (\"OK\")")) -> (T button?=w264:bool)
          }
        }
        n143 = Equal?(x=2.0, y=2.0) -> (x = y?=w203:bool)
        n144 = And(x=w203, y=w202) -> (x .and. y?=w204:bool)
        n145 = case shown="True" w204 {
          frame False {
          }
          frame True {
            n146 = flat-sequence {
              tunnel: "Cycle size" -> [w222]
              tunnel: [w222] -> w220
              tunnel: w220 -> [w225]
              tunnel: [w225] -> w219
              tunnel: w219 -> [w228]
              tunnel: [w228] -> w218
              tunnel: w218 -> [w231]
              tunnel: [w231] -> w217
              tunnel: [w234] -> w221
              tunnel: w217 -> [w234]
              tunnel: [w237] -> w216
              tunnel: w221 -> [w237]
              tunnel: w216 -> [w240]
              tunnel: [w240] -> w214
              tunnel: w214 -> [w243]
              tunnel: [w243] -> w213
              tunnel: w213 -> [w246]
              tunnel: [w246] -> w212
              tunnel: w212 -> [w249]
              tunnel: [w249] -> w211
              tunnel: w211 -> [w261]
              frame #0 {
                n147 = call-poly <vilib>:"Read From Spreadsheet File.vi"() -> ("all rows"=w224:dbl[][])  [unwired: 7 in, 4 out]
                n148 = Reshape Array(w224, w222) -> (→"Air Cyc 1":dbl[])
              }
              frame #1 {
                n149 = call-poly <vilib>:"Read From Spreadsheet File.vi"() -> ("all rows"=w226:dbl[][])  [unwired: 7 in, 4 out]
                n150 = Reshape Array(w226, w225) -> (→"Air Cyc 2":dbl[])
              }
              frame #2 {
                n151 = call-poly <vilib>:"Read From Spreadsheet File.vi"() -> ("all rows"=w230:dbl[][])  [unwired: 7 in, 4 out]
                n152 = Reshape Array(w230, w228) -> (→"HC Cyc 1":dbl[])
              }
              frame #3 {
                n153 = call-poly <vilib>:"Read From Spreadsheet File.vi"() -> ("all rows"=w233:dbl[][])  [unwired: 7 in, 4 out]
                n154 = Reshape Array(w233, w231) -> (→"HC Cyc 2":dbl[])
              }
              frame #4 {
                n155 = call-poly <vilib>:"Read From Spreadsheet File.vi"() -> ("all rows"=w235:dbl[][])  [unwired: 7 in, 4 out]
                n156 = Reshape Array(w235, w234) -> (→"Air Bal":dbl[])
              }
              frame #5 {
                n157 = call-poly <vilib>:"Read From Spreadsheet File.vi"() -> ("all rows"=w239:dbl[][])  [unwired: 7 in, 4 out]
                n158 = Reshape Array(w239, w237) -> (→"HC Bal":dbl[])
              }
              frame #6 {
                n159 = call-poly <vilib>:"Read From Spreadsheet File.vi"() -> ("all rows"=w241:dbl[][])  [unwired: 7 in, 4 out]
                n160 = Reshape Array(w241, w240) -> (→"SO Valve 1":dbl[])
              }
              frame #7 {
                n161 = call-poly <vilib>:"Read From Spreadsheet File.vi"() -> ("all rows"=w244:dbl[][])  [unwired: 7 in, 4 out]
                n162 = Reshape Array(w244, w243) -> (→"SO Valve 2":dbl[])
              }
              frame #8 {
                n163 = call-poly <vilib>:"Read From Spreadsheet File.vi"() -> ("all rows"=w248:dbl[][])  [unwired: 7 in, 4 out]
                n164 = Reshape Array(w248, w246) -> (→"Open/Closed \nLoop":dbl[])
              }
              frame #9 {
                n165 = local read "Open/Closed \nLoop"() -> (w250:dbl[])
                n166 = local read "SO Valve 1"() -> (w252:dbl[])
                n167 = local read "SO Valve 2"() -> (w251:dbl[])
                n168 = local read "HC Cyc 2"() -> (w256:dbl[])
                n169 = local read "HC Cyc 1"() -> (w255:dbl[])
                n170 = local read "Air Cyc 1"() -> (w253:dbl[])
                n171 = local read "Air Cyc 2"() -> (w254:dbl[])
                n172 = local read "HC Bal"() -> (w258:dbl[])
                n173 = local read "Air Bal"() -> (w257:dbl[])
                n174 = Build Array (concatenate)(w249, w253, w254, w255, w256, w257, w258, w252, w251, w250) -> (w259:dbl[])
                n175 = shared-variable "My Computer\\Library 1.lvlib\\Inject_Arrays"(w259) -> ()  [unwired: 1 in, 1 out]
              }
              frame #10 {
                n176 = call-poly <vilib>:"Read From Spreadsheet File.vi"() -> ("all rows"=w262:dbl[][])  [unwired: 7 in, 4 out]
                n177 = Reshape Array(w262, w261) -> (w260:dbl[])
                "Lambda" <- w260
                n178 = shared-variable "My Computer\\Library 1.lvlib\\Inject_Arrays_Lambda"(w260) -> ()  [unwired: 1 in, 1 out]
              }
            }
          }
        }
        n179 = case shown="True" w202 {
          tunnel: w210 -> [_ w269]
          frame False {
          }
          frame True {
            n180 = flat-sequence {
              tunnel: w269 -> [w272]
              tunnel: [w272] -> w268
              tunnel: w268 -> [w276]
              frame #0 {
                n181 = local write "Enum 1"(u16 1 ("Test number")) -> ()
                "Test number" <- "Select Test Type"
              }
              frame #1 {
                n182 = Enqueue Element(queue=w276, element=Control_3."main" ("Enum")) -> (queue out=w274:refnum<queue>)  [unwired: 2 in, 2 out]
                n183 = property on="Stop Test Button" class="Bool"("DisabledEnum"=T11."Enabled" ("Disabled")) -> ()  [unwired: 2 in, 2 out]
                n184 = Enqueue Element(queue=w274, element=Control_3."start test" ("Enum")) -> ()  [unwired: 2 in, 3 out]
              }
            }
          }
        }
      }
      event "Log Test Button": Value Change {
        n185 = event-data() -> ()  [unwired: 1 in, 6 out]
        n186 = property on="File Name" class="Str (strict)"() -> ("Value"=w280:T5)  [unwired: 2 in, 2 out]
        n187 = String Length(string=w280) -> (length=w279:i32)
        n188 = Equal To 0?(x=w279) -> (x = 0?=w278:bool)
        n189 = case shown="True" w278 {
          frame False {
          }
          frame True {
            n190 = One Button Dialog(message="A filename has not been entered!") -> ()  [unwired: 1 in, 1 out]
          }
        }
      }
      event "Stop Test Button": Value Change {
        n191 = event-data() -> ()  [unwired: 1 in, 5 out]
        n192 = flat-sequence {
          tunnel: w287 -> [w289]
          tunnel: [w289] -> w286
          tunnel: [w288] -> w284
          tunnel: w286 -> [w293]
          tunnel: [w292] -> w285
          tunnel: w284 -> [w292]
          tunnel: [w291] -> w283
          tunnel: w285 -> [w297]
          tunnel: w283 -> [w296]
          tunnel: [T11."Disabled and Grayed Out" ("Disabled")] -> w282
          frame #0 {
            n193 = local read "Connected?"() -> (w288:bool)
            n194 = local write "Stop Cmd"(T1 1.0 ("Stop Cmd")) -> ()
          }
          frame #1 {
            n195 = Enqueue Element(queue=w293, element=Control_3."main" ("Enum")) -> (queue out=w291:refnum<queue>)  [unwired: 2 in, 2 out]
          }
          frame #2 {
            n196 = case shown="True" w297 {
              tunnel: w296 -> [w298 w301]
              tunnel: [w298 w300] -> _
              frame False {
              }
              frame True {
                n197 = local write "Connected?"(FALSE ("Connected?")) -> ()
                n198 = Enqueue Element(queue=w301, element=Control_3."Multigas disconnect" ("Enum")) -> (queue out=w300:refnum<queue>)  [unwired: 2 in, 2 out]
              }
            }
          }
        }
        n199 = property on="Stop Test Button" class="Bool"("DisabledEnum"=w282) -> ()  [unwired: 2 in, 2 out]
      }
      event "Stopped?": Value Change {
        n200 = event-data() -> ()  [unwired: 1 in, 5 out]
        n201 = flat-sequence {
          tunnel: w305 -> [w309]
          tunnel: [w308] -> w304
          tunnel: [w307] -> w303
          tunnel: w304 -> [w311]
          tunnel: w303 -> [w310]
          frame #0 {
            n202 = local read "Connected?"() -> (w307:bool)
            n203 = Enqueue Element(queue=w309, element=Control_3."main" ("Enum")) -> (queue out=w308:refnum<queue>)  [unwired: 2 in, 2 out]
          }
          frame #1 {
            n204 = case shown="True" w310 {
              tunnel: w311 -> [_ w312]
              frame False {
              }
              frame True {
                n205 = local write "Connected?"(FALSE ("Connected?")) -> ()
                n206 = Enqueue Element(queue=w312, element=Control_3."Multigas disconnect" ("Enum")) -> ()  [unwired: 2 in, 3 out]
              }
            }
          }
        }
      }
      event "Alarm ack": Value Change {
        # "system alarm - set to off"
        n207 = event-data() -> ()  [unwired: 1 in, 5 out]
        n208 = local write "Acknowledge"(TRUE ("Acknowledge")) -> ()
        n209 = property on="Soft Alarm" class="Bool (strict)"("Value"=FALSE ("Acknowledge")) -> ()  [unwired: 2 in, 2 out]
        n210 = property on="Alarm ack" class="Bool"("DisabledEnum"=T11."Disabled and Grayed Out" ("Disabled")) -> ()  [unwired: 2 in, 2 out]
      }
      event "Purge System": Value Change {
        n211 = event-data() -> ()  [unwired: 1 in, 5 out]
        n212 = flat-sequence {
          tunnel: w319 -> [w321]
          tunnel: [w321] -> w318
          tunnel: w318 -> [w322]
          frame #0 {
            n213 = local write "Enum 1"(u16 4 ("Test number")) -> ()
          }
          frame #1 {
            n214 = Enqueue Element(queue=w322, element=Control_3."start test" ("Enum")) -> ()  [unwired: 2 in, 3 out]
          }
        }
      }
      event "Clear log": Value Change {
        n215 = event-data() -> ()  [unwired: 1 in, 5 out]
        n216 = local write "Table"(string[][] [] ("Table")) -> ()
      }
      event "Adv Settings": Value Change {
        # "To be updated"
        # "SO2 conc\nNOx conc\nCO conc\nHC conc\nBleed ratio N2\nBleed ratio CO2"
        n217 = event-data() -> ()  [unwired: 1 in, 6 out]
        n218 = call "Advanced settings MAX.vi"() -> ("output cluster"=→"output cluster":T2)  [unwired: 1 in]
      }
    }
    "stop 2" <- w40
  }
  n219 = node-c288(nitl_modes."Discard missed periods, maintain original phase" ("Mode")) -> (w10:T12)  [unwired: 4 in]
  n220 = node-c288() -> (w3:T12)  [unwired: 4 in]
  n221 = timed-loop {
    timing: w10 -> [_]
    timing-out: [_] -> w9
    shift-right: [w412] -> _
    shift-left: path "" -> [w371]
    shift-right: [w475] -> _
    shift-left: w4 -> [w515]
    shift-right: [w413] -> _
    shift-left: _ -> [w486]
    shift-right: [w465] -> _
    shift-left: w4 -> [w468]
    shift-right: [w466] -> _
    shift-left: w4 -> [w467]
    shift-right: [w395] -> _
    shift-left: 0 ("t") -> [w394]
    shift-right: [w389] -> _
    shift-left: _ -> [w378]
    shift-right: [w388] -> _
    shift-left: _ -> [w379]
    shift-right: [w387] -> _
    shift-left: _ -> [w380]
    shift-right: [w386] -> _
    shift-left: _ -> [w381]
    shift-right: [w385] -> _
    shift-left: _ -> [w382]
    shift-right: [w384] -> _
    shift-left: _ -> [w383]
    shift-right: [w361] -> _
    shift-left: _ -> [w362]
    shift-right: [w354] -> _
    shift-left: _ -> [w353]
    shift-right: [w342] -> _
    shift-left: _ -> [w341]
    shift-right: [w332] -> _
    shift-left: _ -> [w331]
    stop <- w514 stop-if-true
    w421 = 54321.0 ("y")
    # "Flow Rate Guide"
    # "setting up the header"
    # "Temperature Guide"
    # "0   Flow Rate 1\n1   Flow Rate 2\n     ECM 1\n     ECM 2\n2   CO2 U\n3   CO U\n4   HC U\n5   O2 U\n7   CO2 D\n8   CO D\n9   HC D\n10 O2 D\n12 TC1X\n13 TC2A\n14 TC3Y\n15 TC4B\n16 TC5\n17 TC6\n32 Venturi 1\n33 Venturi 2\n34 Tank\n35 Bearing 1\n36 Bearing 2\n38 Ex A\n39 Ex B\n40 Ex C\n41 Ex D\n     MFC Box\n42 Furnace 1\n43 Furnace 2\n44 NO 1 ?? \n45 Lambda 1\n46 NO 2 ??\n47 Lambda 2"
    n222 = node-c288() -> (→"Finished Late? [i-1]":bool, →"Iteration Duration":i64)  [unwired: 1 in, 1 out]
    n223 = shared-variable "My Computer\\Library 1.lvlib\\DATA"() -> (w513:dbl[])  [unwired: 1 in, 1 out]
    n224 = Type Cast(type=w513, x=w513) -> (*(type *) &x=w523:dbl[])
    n225 = local read "Advanced Logging"() -> (w418:bool)
    n226 = Delete From Array(array=w523, length=4, index=0) -> (deleted portion=w520:dbl[], array with subset deleted=w398:dbl[])
    n227 = call "MKS.vi"("IP Address"="192.168.254.1", "Connect"="MKS") -> ("Emissions"=w375:dbl[])  [unwired: 9 in]
    n228 = call "MKS.vi"("IP Address"="192.168.254.2", "Connect"=FALSE) -> ("Emissions"=w376:dbl[])  [unwired: 9 in]
    n229 = local read "Full system?"() -> (w410:bool)
    n230 = Index Array(array=w375, index=0) -> (element=w425:dbl)
    n231 = Index Array(array=w376, index=0) -> (element=w423:dbl)
    n232 = case shown="False" w418 {
      tunnel: [w545 w596] -> w419
      tunnel: w398 -> [w546 w596]
      tunnel: [w544 "Time\tFlow 1 g/s\tFlow 2 g/s\tECM AFR\tCO2 U %\tCO U %\tHC U ppm\tO2 U %\tNO U ppm\tCO2 D %\tCO D %\tHC D ppm\tO2 D %\tNO D ppm\tTC1X\tTC2A\tTCY\tTC4B\tTC5\tTC6\tTC7\tTC8\tTC9\tTC10\tTC11\tTC12\tTC13\tTC14\tTC15\tTC16\tTC17\tTC18\tTC19\tTC20\tTC Vent 1\tTC Vent 2\tTC Tank\tTC Fan B1\tTC Fan B2\tTC Cab\tTC Ex A\tTC Ex B\tTC Ex C\tTC Ex D\tTC MFC Box\tTC Furn 1\tTC Furn 2\tTank Pressure\tRapidox\tLambda 1\tLambda 2\tNOX 1 ppm\tNOX 2 ppm\tUEGO 1\tUEGO 2" ("Heading string 2")] -> w417
      tunnel: w410 -> [w543 _]
      frame False {
        n233 = case shown="True" w543 {
          tunnel: w546 -> [w561 w576]
          tunnel: [w552 w578] -> w545
          tunnel: ["Time\tFlow 1 g/s\tCO2 U %\tCO U %\tHC U ppm\tO2 U %\tNO U ppm\tCO2 D %\tCO D %\tHC D ppm\tO2 D %\tNO D ppm\tTC1X\tTC2A\tTCY\tTC4B\tTC5\tTC6\tTC7\tTC8\tRapidox\tLambda 1\tLambda 2\tNOX 1 ppm\tNOX 2 ppm\tUEGO 1\tUEGO 2" ("Heading string 2") "Time\tFlow 1 g/s\tFlow 2 g/s\tCO2 U %\tCO U %\tHC U ppm\tO2 U %\tNO U ppm\tCO2 D %\tCO D %\tHC D ppm\tO2 D %\tNO D ppm\tTC1X\tTC2A\tTCY\tTC4B\tTC5\tTC6\tTC7\tTC8\tRapidox\tLambda 1\tLambda 2\tNOX 1 ppm\tNOX 2 ppm\tUEGO 1\tUEGO 2" ("Heading string 2")] -> w544
          frame False {
            n234 = Delete From Array(array=w561, length=21, index=0) -> (deleted portion=w548:dbl[], array with subset deleted=w560:dbl[])
            n235 = Index Array(array=w560, index #1=47 ("index"), index #2=48 ("index"), index #3=49 ("index"), index #4=50 ("index"), index #5=51 ("index"), index #6=52 ("index"), index #7=53 ("index")) -> (element #1=w559:dbl, element #2=w558:dbl, element #3=w557:dbl, element #4=w556:dbl, element #5=w555:dbl, element #6=w554:dbl, element #7=w553:dbl)
            n236 = Delete From Array(array=w548, length=1, index=2) -> (array with subset deleted=w547:dbl[])  [unwired: 1 out]
            n237 = Build Array (concatenate)(w547, w559, w558, w557, w556, w555, w554, w553) -> (w552:dbl[])
          }
          frame True {
            n238 = Delete From Array(array=w576, length=21, index=0) -> (deleted portion=w573:dbl[], array with subset deleted=w577:dbl[])
            n239 = Index Array(array=w577, index #1=47 ("index"), index #2=48 ("index"), index #3=49 ("index"), index #4=50 ("index"), index #5=51 ("index"), index #6=52 ("index"), index #7=53 ("index")) -> (element #1=w585:dbl, element #2=w584:dbl, element #3=w583:dbl, element #4=w582:dbl, element #5=w581:dbl, element #6=w580:dbl, element #7=w579:dbl)
            n240 = Delete From Array(array=w573, length=2, index=1) -> (array with subset deleted=w571:dbl[])  [unwired: 1 out]
            n241 = Build Array (concatenate)(w571, w585, w584, w583, w582, w581, w580, w579) -> (w578:dbl[])
          }
        }
      }
      frame True {
        (unwired) "Time\tFlow 1 g/s\tFlow 2 g/s\tECM AFR\tCO2 U %\tCO U %\tHC U ppm\tO2 U %\tNO U ppm\tCO2 D %\tCO D %\tHC D ppm\tO2 D %\tNO D ppm\tTC1X\tTC2A\tTCY\tTC4B\tTC5\tTC6\tTC7\tTC8\tTC9\tTC10\tTC11\tTC12\tTC13\tTC14\tTC15\tTC16\tTC17\tTC18\tTC19\tTC20\tTC Vent 1\tTC Vent 2\tTC Fan B1\tTC Fan B2\tTC Cab\tTC Ex A\tTC Ex B\tTC Ex C\tTC Ex D\tTC Furn 1\tTC Furn 2\tNOX 1 ppm\tNLambda 1\tNOX 2 ppm\tNLambda 2\tEGO 1\tEGO 2\tEGO 3\tEGO 4\tCO2 U %\tCO U %\tHC U ppm\tO2 U %\tNO U ppm\tCO2 D %\tCO D %\tHC D ppm\tO2 D %\tNO D ppm\r\n" ("Heading string 2")
      }
    }
    n242 = Not Equal?(x=w425, y=w421) -> (x != y?=w424:bool)
    n243 = Not Equal?(x=w421, y=w423) -> (x != y?=w422:bool)
    n244 = Index Array(array=w520) -> (element #1=w413:dbl, element #2=w492:dbl, element #3=w415:dbl, element #4=w485:dbl)  [unwired: 4 in]
    "Error" <- w415
    n245 = case shown="True" w424 {
      tunnel: [w602 w613] -> w373
      tunnel: w376 -> [w601 w612]
      tunnel: w375 -> [_ w611]
      tunnel: w422 -> [w600 w610]
      tunnel: [w599 w607] -> w420
      frame False {
        n246 = case shown="False" w600 {
          tunnel: [dbl[] [54321.0] w606] -> w602
          tunnel: w601 -> [_ w606]
          tunnel: ["\r\n" ("Heading string 2") "\tNO\tNO2 (150)\tNO2 (2000)\tN2O\tNH3 (300)\tNH3 (3000)\tHNCO (400)\tH2O\tCO2\tCO (500)\tCO (1)\tCH4 (250)\tCH4 (3000)\tNOxP\tPropane\r\n" ("Heading string 2")] -> w597
          frame False {
          }
          frame True {
          }
        }
        n247 = Build Array(" " ("Heading string 2"), w597) -> (w599:string[])
      }
      frame True {
        n248 = case shown="True" w610 {
          tunnel: [w615 w619] -> w613
          tunnel: w612 -> [_ w618]
          tunnel: w611 -> [w615 w617]
          tunnel: ["\rn" ("Heading string 2") "\tNO\tNO2 (150)\tNO2 (2000)\tN2O\tNH3 (300)\tNH3 (3000)\tHNCO (400)\tH2O\tCO2\tCO (500)\tCO (1)\tCH4 (250)\tCH4 (3000)\tNOxP\tPropane\r" ("Heading string 2")] -> w608
          frame False {
          }
          frame True {
            n249 = Build Array (concatenate)(w617, w618) -> (w619:dbl[])
          }
        }
        n250 = Build Array("\tNO\tNO2 (150)\tNO2 (2000)\tN2O\tNH3 (300)\tNH3 (3000)\tHNCO (400)\tH2O\tCO2\tCO (500)\tCO (1)\tCH4 (250)\tCH4 (3000)\tNOxP\tPropane" ("Heading string 2"), w608) -> (w607:string[])
      }
    }
    n251 = To Unsigned Long Integer(number=w485) -> (unsigned 32bit integer=w484:u32)
    n252 = Number To Boolean Array(number=w484) -> (Boolean array=w503:bool[])
    n253 = Index Array(array=w503) -> (element #2=w501:bool, element #3=w500:bool, element #4=w481:bool, element #5=→"ExtAnUp":bool, element #6=→"ExtAnDn":bool)  [unwired: 6 in, 1 out]
    "Extractor Fan On" <- w481
    n254 = case shown="2" w492 {
      tunnel: [w639 TRUE FALSE] -> w491
      tunnel: [w640 FALSE TRUE] -> w490
      frame 0, Default {
        n255 = local read "Pass"() -> (w640:bool)
        n256 = local read "Fail"() -> (w639:bool)
      }
      frame 1 {
      }
      frame 2 {
      }
    }
    "Pass" <- w490
    "Fail" <- w491
    n257 = Or(x=w501, y=w500) -> (x .or. y?=→"Doors Open":bool)
    n258 = Not(x=w481) -> (.not. x?=→"Doors Unlocked":bool)
    n259 = Less?(x=w413, y=w486) -> (x < y?=w483:bool)
    n260 = Path To String(path="File Path") -> (string=w479:string)
    n261 = local read "Connected"() -> (w482:bool)
    n262 = Concatenate Strings(w479, "\\" ("string"), "File Name") -> (w428:string)
    n263 = call "Mexa_7170.vi"("String 1 In"=w382, "Connect"="7170", "connection ID 1 In"=w381, "error out 1 In"=w380, "connection ID 2 In"=w379, "error out 2 In"=w378, "Time In"=w383) -> ("Emissions"=w374:dbl[], "String 1 Out"=w385:string, "connection ID 1 Out"=w386:refnum<k5>, "error 1 out"=w387:errorcluster, "connection ID 2 Out"=w388:refnum<k16>, "Time Out"=w384:i16, "error 2 out"=w389:errorcluster)  [unwired: 2 in]
    "Emissions" <- w374
    n264 = Build Array (concatenate)(w374, w373) -> (w372:dbl[])
    n265 = And(x=w482, y=w483) -> (x .and. y?=w474:bool)
    n266 = local write "Stopped?"(w474) -> ()
    n267 = Equal To 0?(x=w415) -> (x = 0?=w416:bool)
    n268 = Equal To 0?(x=w413) -> (x = 0?=w414:bool)
    n269 = Build Array (concatenate)(w419, w372) -> (w516:dbl[])
    n270 = Equal?(x=w413, y=2.0) -> (x = y?=w436:bool)
    n271 = String To Path(string=w428) -> (path=w476:path)
    n272 = Build Array(w416, w414) -> (w497:bool[])
    n273 = Equal?(x=w413, y=3.0) -> (x = y?=w433:bool)
    n274 = Equal?(x=w413, y=4.0) -> (x = y?=w431:bool)
    n275 = Boolean Array To Number(Boolean array=w497) -> (number=w496:u32)
    n276 = Not Equal?(x=w476, y=w371) -> (x != y?=w525:bool)
    n277 = Compound Arithmetic op=OR(w436, w433, w431) -> (w435:bool)
    n278 = local read "Log Test Button"() -> (w429:bool)
    n279 = case shown="2" w496 {
      tunnel: [w664 w665 w670 w672] -> w498
      tunnel: [w664 w665 w670 w672] -> w495
      tunnel: [w664 w665 w670 w672] -> w494
      tunnel: [w664 w665 w668 w672] -> w493
      tunnel: [T11."Enabled" ("Disabled") T11."Enabled" ("Disabled") w668 w672] -> _
      tunnel: [FALSE FALSE FALSE TRUE] -> w473
      frame 0, Default {
        w664 = T11."Disabled and Grayed Out" ("Disabled")
      }
      frame 1 {
        w665 = T11."Disabled and Grayed Out" ("Disabled")
      }
      frame 2 {
        w668 = T11."Enabled" ("Disabled")
        w670 = T11."Disabled and Grayed Out" ("Disabled")
      }
      frame 3 {
        w672 = T11."Enabled" ("Disabled")
        (unwired) T11."Disabled and Grayed Out" ("Disabled")
      }
    }
    n280 = for {
      tunnel: w516 -> [w680] mode=indexing
      tunnel: [w679] -> w527 mode=indexing
      n281 = Number To Fractional String(number=w680, precision (6)=i16 3) -> (F-format string=w679:string)  [unwired: 2 in]
    }
    n282 = Select(t=w476, s=w525, f=w371) -> (s? t:f=w526:path)
    n283 = And(x=w429, y=w435) -> (x .and. y?=w542:bool)
    "Log?" <- w542
    n284 = case shown="True" w525 {
      tunnel: w526 -> [w673 w678]
      tunnel: [w673 w677] -> w524
      tunnel: w420 -> [_ w675]
      tunnel: w417 -> [_ w674]
      frame False {
      }
      frame True {
        n285 = Build Array (concatenate)(w674, w675) -> (w676:string[])
        n286 = call-poly <vilib>:"Write To Spreadsheet File.vi"("1D data"=w676, "file path (dialog if empty)"=w678) -> ("new file path (Not A Path if cancelled)"=w677:path)  [unwired: 6 in]
      }
    }
    n287 = Equal?(x=w413, y=0.0) -> (x = y?=w462:bool)
    n288 = case shown="5" w413 {
      tunnel: [w626 w629 w631 w633 TRUE FALSE] -> w489
      tunnel: [w626 TRUE TRUE TRUE w635 w637] -> w488
      tunnel: [TRUE w629 w631 w633 w635 w637] -> w487
      frame 0, Default {
        w626 = FALSE
      }
      frame 1 {
        w629 = FALSE
      }
      frame 2 {
        w631 = FALSE
      }
      frame 3 {
        w633 = FALSE
      }
      frame 4 {
        w635 = FALSE
        n289 = local write "Stop Cmd"(T1 0.0 ("Stop Cmd")) -> ()
      }
      frame 5 {
        w637 = FALSE
      }
    }
    "Cool Down" <- w489
    "Test In Progress" <- w488
    "Standby" <- w487
    n290 = property class="VI"("Front Panel.Closeable"=w473) -> ()  [unwired: 2 in, 2 out]
    n291 = property on="Start Test Button" class="Bool"("DisabledEnum"=w498) -> ()  [unwired: 2 in, 2 out]
    n292 = property on="Execute Leak Test Button" class="Bool"("DisabledEnum"=w495) -> ()  [unwired: 2 in, 2 out]
    n293 = property on="Compile Test Button" class="Bool"("DisabledEnum"=w494) -> ()  [unwired: 2 in, 2 out]
    n294 = property on="Purge System" class="Bool"("DisabledEnum"=w493) -> ()  [unwired: 2 in, 2 out]
    n295 = Index Array(array=w372, index #1=0 ("index"), index #2=1 ("index"), index #3=2 ("index"), index #4=3 ("index")) -> ()  [unwired: 4 out]
    n296 = local read "Full system?"() -> (w463:bool)
    n297 = Not Equal To 0?(x=w415) -> (x != 0?=w518:bool)
    n298 = Not Equal?(x=w415, y=w515) -> (x != y?=w517:bool)
    n299 = case shown="True" w542 {
      tunnel: w524 -> [w684 w692]
      tunnel: [w684 w704] -> w412
      tunnel: w527 -> [_ w700]
      tunnel: w468 -> [_ w693]
      tunnel: w467 -> [w683 w688]
      tunnel: [w683 w690] -> w466
      tunnel: [w682 w689] -> w465
      frame False {
        n300 = local read "Log interval (seconds)"() -> (w682:T1)
      }
      frame True {
        n301 = Get Date/Time In Seconds() -> (seconds since 1Jan1904=w701:timestamp)
        n302 = Decrement(x=w693) -> (x-1=w694:T1)
        n303 = Less Than 0?(x=w694) -> (x < 0?=w695:bool)
        n304 = Equal To 0?(x=w694) -> (x = 0?=w696:bool)
        n305 = Build Array(w695, w696) -> (w697:bool[])
        n306 = Path To String(path=w692) -> (string=w687:string)
        "File name" <- w687
        n307 = Format Date/Time String(time format string (%c)="%d/%m/%y %H:%M:%S", seconds (now)=w701) -> (date/time string=w702:string)  [unwired: 1 in]
        n308 = Boolean Array To Number(Boolean array=w697) -> (number=w698:u32)
        n309 = case shown="2" w698 {
          tunnel: w693 -> [w711 w712 _]
          tunnel: [w710 w712 w715] -> w689
          tunnel: w687 -> [w709 w714 w718]
          tunnel: [w706 w714 w716] -> w691
          tunnel: [w705 w713 w717] -> w690
          tunnel: w688 -> [w705 w713 w721]
          frame 0, Default {
            n310 = Number To Decimal String(number=w705) -> (decimal integer string=w707:string)  [unwired: 1 in]
            n311 = call <vilib>:"Space Constant.vi"() -> ("String"=w708:string)
            n312 = Decrement(x=w711) -> (x-1=w710:T1)
            n313 = Concatenate Strings(w709, w708, w707) -> (w706:string)
          }
          frame 1 {
          }
          frame 2 {
            n314 = Increment(x=w721) -> (x+1=w717:dbl)
            n315 = local read "Log interval (seconds)"() -> (w715:T1)
            n316 = Number To Decimal String(number=w717) -> (decimal integer string=w719:string)  [unwired: 1 in]
            n317 = call <vilib>:"Space Constant.vi"() -> ("String"=w720:string)
            n318 = Concatenate Strings(w718, w720, w719) -> (w716:string)
          }
        }
        n319 = Build Array (concatenate)(w702, w700) -> (w686:string[])
        n320 = String To Path(string=w691) -> (path=w685:path)
        n321 = call-poly <vilib>:"Write To Spreadsheet File.vi"("append to file? (new file:F)"=TRUE, "1D data"=w686, "file path (dialog if empty)"=w685) -> ("new file path (Not A Path if cancelled)"=w704:path)  [unwired: 5 in]
      }
    }
    n322 = And(x=w518, y=w517) -> (x .and. y?=w519:bool)
    n323 = Index Array(array=w398, index #1=0 ("index"), index #2=1 ("index"), index #3=4 ("index"), index #4=5 ("index"), index #5=7 ("index"), index #6=9 ("index"), index #7=10 ("index"), index #8=12 ("index"), index #9=6 ("index"), index #10=11 ("index"), index #11=14 ("index"), index #12=15 ("index"), index #13=16 ("index"), index #14=17 ("index"), index #15=18 ("index"), index #16=19 ("index"), index #17=34 ("index"), index #18=35 ("index"), index #19=36 ("index"), index #20=37 ("index"), index #21=38 ("index"), index #22=40 ("index"), index #23=41 ("index"), index #24=42 ("index"), index #25=43 ("index"), index #26=45 ("index"), index #27=46 ("index"), index #28=51 ("index"), index #29=52 ("index"), index #30=49 ("index"), index #31=50 ("index"), index #32=2 ("index"), index #33=3 ("index")) -> (element #1=w397:dbl, element #2=w396:dbl, element #3=w460:dbl, element #4=w459:dbl, element #5=w409:dbl, element #6=w408:dbl, element #7=w407:dbl, element #8=w406:dbl, element #9=w405:dbl, element #10=w404:dbl, element #26=→"Furnace temp 1":dbl, element #27=→"Furnace temp 2":dbl, element #28=w439:dbl, element #29=w411:dbl)  [unwired: 19 out]
    n324 = Build Array(w463, w462) -> (w464:bool[])
    n325 = case shown="True" w519 {
      tunnel: w415 -> [w646 w657]
      tunnel: w517 -> [w649 _]
      tunnel: [w645 w657] -> w475
      frame False {
        n326 = Equal To 0?(x=w646) -> (x = 0?=w650:bool)
        n327 = And(x=w650, y=w649) -> (x .and. y?=w648:bool)
        n328 = case shown="True" w648 {
          frame False {
          }
          frame True {
            w653 = FALSE ("Ack hard alarm!")
            n329 = property on="Hard Alarm" class="Bool (strict)"("Value"=w653) -> ()  [unwired: 2 in, 2 out]
            n330 = property on="System Alarm" class="Bool (strict)"("Value"=w653) -> ()  [unwired: 2 in, 2 out]
          }
        }
        n331 = case shown="False" "Acknowledge" {
          tunnel: [w651 0.0 ("Numeric")] -> w645
          tunnel: w646 -> [w651 _]
          frame False {
          }
          frame True {
          }
        }
      }
      frame True {
        n332 = local read "Table"() -> (w660:string[][])
        n333 = call "Error list.vi"("Error code"=w657, "Error array in"=w660) -> ("Hard alarm?"=w654:bool, "Error array out"=w659:string[][])  [unwired: 8 in]
        "Hard Alarm" <- w654
        "System Alarm" <- w654
        n334 = Not(x=w654) -> (.not. x?=w655:bool)
        "Soft Alarm" <- w655
        n335 = case shown="True" w655 {
          frame False {
          }
          frame True {
            n336 = property on="Alarm ack" class="Bool"("DisabledEnum"=T11."Enabled" ("Disabled")) -> ()  [unwired: 2 in, 2 out]
          }
        }
        n337 = local write "Table"(w659) -> ()
        n338 = local write "Acknowledge"(FALSE ("Acknowledge")) -> ()
        n339 = property on="Tab Control" class="TabCtl (strict)"("Value"=6) -> ()  [unwired: 2 in, 2 out]
      }
    }
    n340 = Boolean Array To Number(Boolean array=w464) -> (number=w461:u32)
    n341 = case shown="1" w461 {
      tunnel: w397 -> [w621 w623 _ _]
      tunnel: w396 -> [_ w622 _ _]
      tunnel: [w621 w623 w624 w625] -> _
      tunnel: [0.0 ("y") w622 w624 w625] -> _
      frame 0, Default {
      }
      frame 1 {
      }
      frame 2 {
        w624 = 0.0 ("y")
      }
      frame 3 {
        w625 = 0.0 ("y")
      }
    }
    n342 = call "Flow_Guide-plot.vi"("Time In"=w362, "Temperature Sync"="Flow Sync", "Temp Band % (e.g. 1%=1.01)"="Flow Band %", "Mean(Off)/Interval(On)"="Mean(Off)/Interval(On) 2", "Guide"="FlowGuide") -> ("Graph 2"=w359:dbl, "Graph 1"=w360:dbl, "Time out"=w361:i32)  [unwired: 4 in]
    n343 = call "Lambda_Guide-plot.vi"("Time In"=w353, "Temperature Sync"="Lambda Sync", "Temp Band % (e.g. 1%=1.01)"="Lambda Band %", "Mean(Off)/Interval(On)"="Mean(Off)/Interval(On) 3", "Guide"="Lambda Guide") -> ("Graph 2"=w347:dbl, "Graph 1"=w348:dbl, "Time out"=w354:i32)  [unwired: 4 in]
    n344 = Merge Signals(w360, w359) -> (→"Flow Rate (g/s)":dynamicdata)
    n345 = Merge Signals(w460, w459, w409, w408, w407, w406) -> (→"M584L Upstream & Downstream":dynamicdata)
    n346 = Merge Signals(w439, w411) -> (→"NO Concentration (ppm)":dynamicdata)
    n347 = Merge Signals(w348, w347) -> (→"Lambda":dynamicdata)
    n348 = call "Heat_Exch_Guide-plot.vi"("Time In"=w341, "Temperature Sync"="Heat Sync", "Temp Band % (e.g. 1%=1.01)"="Heat Band %", "Mean(Off)/Interval(On)"="Mean(Off)/Interval(On) 4", "TempGuide"="Heat Guide") -> ("Graph 4"=w343:dbl, "Graph 3"=w344:dbl, "Graph 2"=w345:dbl, "Graph 1"=w346:dbl, "Time out"=w342:i32)  [unwired: 2 in]
    n349 = local read "MKS HC"() -> (w401:dbl)
    n350 = Merge Signals(w405, w404, w401) -> (→"HC Concentration (ppm)":dynamicdata)
    n351 = Merge Signals(w346, w345, w344, w343) -> (→"Heat Exchanger Temperatures (°C)":dynamicdata)
    n352 = call "Temp_Guide-plot.vi"("Time In"=w394, "Temperature Sync"="Temperature Sync", "Temp Band % (e.g. 1%=1.01)"="Temp Band %", "Mean(Off)/Interval(On)"="Mean(Off)/Interval(On)", "TempGuide"="TempGuide") -> ("Graph 4"=w355:dbl, "Graph 3"=w356:dbl, "Graph 2"=w357:dbl, "Graph 1"=w358:dbl, "Time out"=w395:i32)  [unwired: 2 in]
    n353 = local read "stop 2"() -> (w514:bool)
    n354 = Merge Signals(w358, w357, w356, w355) -> (→"Sample Temperatures (°C)":dynamicdata)
    n355 = call "System_Guide-plot.vi"("Time In"=w331, "Temperature Sync"="System Sync", "Temp Band % (e.g. 1%=1.01)"="System Band", "Mean(Off)/Interval(On)"="Mean(Off)/Interval(On) 5", "TempGuide"="System Guide") -> ("Graph 4"=w336:dbl, "Graph 3"=w335:dbl, "Graph 2"=w334:dbl, "Graph 1"=w333:dbl, "Time out"=w332:i32)  [unwired: 2 in]
    n356 = Merge Signals(w333, 1372.0, w334, w335, w336) -> (→"System Temperatures (°C)":dynamicdata)
    n357 = node-c288() -> ()  [unwired: 1 in, 1 out]
  }
  n358 = timed-loop {
    timing: w3 -> [_]
    timing-out: [_] -> w2
    stop <- _ stop-if-true
    n359 = node-c288() -> ()  [unwired: 1 in, 1 out]
    n360 = shared-variable "My Computer\\Library 1.lvlib\\DATA_2"() -> (w733:dbl[])  [unwired: 1 in, 1 out]
    n361 = Add(x=0 ("index"), y="MFC Number") -> (x+y=w735:i32)
    n362 = Add(x="MFC Number", y=6) -> (x+y=w734:i32)
    n363 = call "MKS.vi"("IP Address"="192.168.254.2" ("IP_ADD [127.0.0.1]"), "Connect"="MKS") -> ("Emissions"=w726:dbl[])  [unwired: 9 in]
    n364 = Build Array (concatenate)(w733, w726) -> (w732:dbl[])
    n365 = for {
      tunnel: w732 -> [w757] mode=indexing
      tunnel: [w756] -> w743 mode=indexing
      n366 = Number To Fractional String(number=w757, precision (6)=i16 3) -> (F-format string=w756:string)  [unwired: 2 in]
    }
    n367 = Index Array(array=w733, index #1=w735, index #2=w734) -> (element #1=w740:dbl, element #2=w739:dbl)
    n368 = Get Date/Time In Seconds() -> (seconds since 1Jan1904=w746:timestamp)
    n369 = local read "File name"() -> (w750:string)
    n370 = Index Array(array=w726, index="HC Index") -> (element=→"MKS HC":dbl)
    n371 = Format Date/Time String(time format string (%c)="%d/%m/%y %H:%M:%S", seconds (now)=w746) -> (date/time string=w744:string)  [unwired: 1 in]
    n372 = Concatenate Strings(w750, "_MFC" ("string")) -> (w748:string)
    n373 = Build Array (concatenate)(w744, w743) -> (w742:string[])
    n374 = String To Path(string=w748) -> (path=w745:path)
    n375 = local read "Log?"() -> (w741:bool)
    n376 = case shown="True" w741 {
      tunnel: w745 -> [w751 w754]
      tunnel: [w751 w752] -> _
      tunnel: w742 -> [_ w753]
      frame False {
      }
      frame True {
        n377 = call-poly <vilib>:"Write To Spreadsheet File.vi"("append to file? (new file:F)"=TRUE, "1D data"=w753, "file path (dialog if empty)"=w754) -> ("new file path (Not A Path if cancelled)"=w752:path)  [unwired: 5 in]
      }
    }
    n378 = Merge Signals(w740, w739) -> (→"MFC Setpoint/Delivery":dynamicdata)
    n379 = node-c288() -> ()  [unwired: 1 in, 1 out]
  }
  n380 = while {
    tunnel: w38 -> [w765]
    tunnel: w22 -> [w763]
    tunnel: w24 -> [w762]
    tunnel: [FALSE ("stop 2")] -> w12
    stop <- w766 stop-if-true
    n381 = Dequeue Element(queue=w765) -> (element=w764:T10)  [unwired: 2 in, 3 out]
    n382 = case shown="\"main\", Default" w764 {
      tunnel: w763 -> [_ _ _ w821 w832 w868 w902 _ _ _ _ _ _ _ w1265 _ _ _ _ _ _ _]
      tunnel: w762 -> [_ _ _ _ _ _ _ _ w915 w930 w985 w1030 _ _ _ _ _ _ _ _ _ _]
      frame "main", Default {
        # "20"
        # "25"
        # "30"
        # "15"
        # "10"
        # "5"
        # "0"
        # "30"
        # "25"
        # "20"
        # "15"
        # "10"
        # "5"
        # "0"
        # "Output Cluster\n\n0 NOx Conc\n1 CO conc %\n2 HC conc %\n3 Bleed H2O \n4 Bleed CO2\n5 Bleed N2 \n6 lambda P\n7 lambda I\n8 lambda D\n9 purge duration\n10 Target furnace lambda\n11 HC reaction ct\n12 Full system\n13 Log interval\n14 MKS 1\n15 MKS 2"
        n383 = local read "output cluster"() -> (w795:T2)
        n384 = Unbundle(w795) -> ("NOx Concentration (ppm)"=w781:T1, "CO concentration %"=w780:T1, "HC concentration %"=w779:T1, "Bleed H2O %"=w778:T1, "Bleed CO2 %"=w777:T1, "Bleed N2 %"=w792:T1, "lambda P"=w791:T1, "lambda I"=w790:T1, "lambda D"=w793:T1, "Purge duration (seconds)"=w794:T1, "Target furnace lambda"=w786:T1, "HC reaction constant"=w785:T1, w787:i16, "Log interval (HRS)"=→"Log interval (seconds)":T1, w774:i16, w772:i16, "Advanced Logging"=→"Advanced Logging":bool, "Cycle Length (Hours)"=w770:T1, "Heat Load Control"=w769:bool, w767:T1[])
        "MKS 1" <- w774
        "MKS 2" <- w772
        n385 = local read "Test Flow Rate(g/s)"() -> (w807:T1)
        n386 = local read "Test number"() -> (w812:u16)
        n387 = local read "Inlet LAMBDA"() -> (w799:T1)
        n388 = local read "NO ppm Loff"() -> (w797:T1)
        n389 = local read "NO:CO Ratio"() -> (w796:T1)
        n390 = local read "Inlet O2 (%)"() -> (w798:T1)
        n391 = local read "Connected"() -> (w801:bool)
        n392 = Boolean To (0,1)(Boolean=w769) -> (0, 1=w768:i16)
        n393 = Boolean To (0,1)(Boolean=w801) -> (0, 1=w784:i16)
        n394 = Build Array (concatenate)("Stop Cmd", w812, w807, "Test Start Temperature (°C)", "Test Stop temperature (°C)", "Furnace Ramp Rate (°C/min)", w799, w798, "Inlet LAMBDA Rich", "Inlet LAMBDA Lean", "Inlet Temperature (°C)", "NO ppm SW", w797, w796, "Temperature Limit (°C)", w784, "Inlet temp Age", "Flow rate Age", w781, w780, w779, w778, w777, w792, w791, w790, w793, w794, w786, w785, w787, w770, w768, w767) -> (w803:T1[])
        n395 = Not Equal To 0?(x=w787) -> (x != 0?=→"Full system?":bool)
        n396 = shared-variable "My Computer\\Library 1.lvlib\\Control Variables"(w803) -> ()  [unwired: 1 in, 1 out]
        n397 = Not Equal To 0?(x=w774) -> (x != 0?=w775:bool)
        n398 = Not Equal To 0?(x=w772) -> (x != 0?=w773:bool)
        n399 = Or(x=w775, y=w773) -> (x .or. y?=→"Connected":bool)
      }
      frame "start test" {
        w813 = FALSE
        n400 = property on="Pass" class="Bool (strict)"("Value"=w813) -> ()  [unwired: 2 in, 2 out]
        n401 = property on="Fail" class="Bool (strict)"("Value"=w813) -> ()  [unwired: 2 in, 2 out]
        n402 = local write "Pass"(w813) -> ()
        n403 = local write "Fail"(w813) -> ()
        n404 = shared-variable "My Computer\\Library 1.lvlib\\Enum 1"("Enum 1") -> ()  [unwired: 1 in, 1 out]
      }
      frame "clear table 1" {
        n405 = property on="Sub-Cycle Name" class="Str (strict)"("Value"="" ("Subcycle name")) -> ()  [unwired: 2 in, 2 out]
        n406 = local write "Sub-Cycle Pattern"(string[][] [["", "0", "", "", "", "", "", "", "", "", "", "", ""], ["", "", "", "", "", "", "", "", "", "", "", "", ""], ["", "", "", "", "", "", "", "", "", "", "", "", ""], ["", "", "", "", "", "", "", "", "", "", "", "", ""], ["", "", "", "", "", "", "", "", "", "", "", "", ""], ["", "", "", "", "", "", "", "", "", "", "", "", ""], ["", "", "", "", "", "", "", "", "", "", "", "", ""], ["", "", "", "", "", "", "", "", "", "", "", "", ""], ["", "", "", "", "", "", "", "", "", "", "", "", ""], ["", "", "", "", "", "", "", "", "", "", "", "", ""], ["", "", "", "", "", "", "", "", "", "", "", "", ""], ["", "", "", "", "", "", "", "", "", "", "", "", ""], ["", "", "", "", "", "", "", "", "", "", "", "", ""], ["", "", "", "", "", "", "", "", "", "", "", "", ""], ["", "", "", "", "", "", "", "", "", "", "", "", ""], ["", "", "", "", "", "", "", "", "", "", "", "", ""], ["", "", "", "", "", "", "", "", "", "", "", "", ""], ["", "", "", "", "", "", "", "", "", "", "", "", ""], ["", "", "", "", "", "", "", "", "", "", "", "", ""], ["", "", "", "", "", "", "", "", "", "", "", "", ""], ["", "", "", "", "", "", "", "", "", "", "", "", ""], ["", "", "", "", "", "", "", "", "", "", "", "", ""], ["", "", "", "", "", "", "", "", "", "", "", "", ""], ["", "", "", "", "", "", "", "", "", "", "", "", ""], ["", "", "", "", "", "", "", "", "", "", "", "", ""], ["", "", "", "", "", "", "", "", "", "", "", "", ""], ["", "", "", "", "", "", "", "", "", "", "", "", ""], ["", "", "", "", "", "", "", "", "", "", "", "", ""], ["", "", "", "", "", "", "", "", "", "", "", "", ""], ["", "", "", "", "", "", "", "", "", "", "", "", ""], ["", "", "", "", "", "", "", "", "", "", "", "", ""]]) -> ()
        n407 = local write "Flag1"(FALSE) -> ()
      }
      frame "update list 1" {
        n408 = String To Path(string=w821) -> (path=w820:path)
        n409 = List Folder(path=w820, pattern="*.eyes") -> (filenames=w819:string[])  [unwired: 2 in, 3 out]
        n410 = property on="Sub-Cycle List" class="LstBox (strict)"("Item Names"=w819) -> ()  [unwired: 2 in, 2 out]
      }
      frame "save subc" {
        w825 = ".eyes" ("string")
        n411 = local read "Sub-Cycle Name"() -> (w824:T5)
        n412 = String To Path(string=w832) -> (path=w837:path)
        n413 = Equal?(x=w824, y="") -> (x = y?=w829:bool)
        n414 = List Folder(path=w837, pattern="*.eyes" ("string")) -> (filenames=w836:string[])  [unwired: 2 in, 3 out]
        n415 = Concatenate Strings(w824, w825) -> (w823:string)
        n416 = Concatenate Strings(w832, w824, w825) -> (w838:string)
        n417 = Search 1D Array(1D array=w836, element=w823) -> (index of element=w835:i32)  [unwired: 1 in]
        n418 = case shown="True" w829 {
          tunnel: [TRUE FALSE] -> w828
          frame False {
          }
          frame True {
            n419 = One Button Dialog(message="Insert file name!") -> ()  [unwired: 1 in, 1 out]
          }
        }
        n420 = String To Path(string=w838) -> (path=w831:path)
        n421 = Equal?(x=w835, y=-1) -> (x = y?=w833:bool)
        n422 = case shown="False" w833 {
          selector: w833 -> [_ w844]
          tunnel: [w842 w844] -> w827
          frame False {
            n423 = Two Button Dialog(message="A file with this name already exists!\nDo you want to overwrite?") -> (T button?=w842:bool)  [unwired: 2 in]
          }
          frame True {
          }
        }
        n424 = And(x=w827, y=w828) -> (x .and. y?=w826:bool)
        n425 = case shown="True" w826 {
          tunnel: w831 -> [_ w849]
          frame False {
          }
          frame True {
            n426 = local read "Sub-Cycle Pattern"() -> (w848:string[][])
            n427 = call "Table check.vi"("Input table"=w848) -> ("Incomplete?"=w846:bool, "Length"=w847:i32)  [unwired: 9 in]
            n428 = case shown="False" w846 {
              tunnel: w848 -> [w857 _]
              tunnel: w849 -> [w856 _]
              tunnel: w847 -> [w855 _]
              tunnel: string[] [] -> [w854 _]
              frame False {
                n429 = for {
                  N: w855 -> [_]
                  tunnel: w857 -> [w864]
                  shift-right: [w861] -> w853
                  shift-left: w854 -> [w862]
                  i -> [w863]
                  n430 = Index Array(array=w864, index (row)=w863) -> (element=w860:string[])  [unwired: 1 in]
                  n431 = Delete From Array(array=w860, index=0) -> (array with subset deleted=w859:string[])  [unwired: 1 in, 1 out]
                  n432 = Build Array (concatenate)(w862, w859) -> (w861:string[])
                }
                n433 = Build Array (concatenate)("SubCycle Data File for EYECAT - do not modify", w853) -> (w851:string[])
                n434 = call-poly <vilib>:"Write To Spreadsheet File.vi"("1D data"=w851, "file path (dialog if empty)"=w856) -> ()  [unwired: 6 in, 1 out]
              }
              frame True {
                n435 = One Button Dialog(message="The table is incomplete!\nplease review and save again!") -> ()  [unwired: 1 in, 1 out]
              }
            }
            n436 = local write "Flag1"(FALSE) -> ()
          }
        }
      }
      frame "load subc" {
        n437 = local read "Flag1"() -> (w869:bool)
        n438 = case shown="True" w869 {
          tunnel: [w896 w898] -> w867
          tunnel: w868 -> [w896 w898]
          tunnel: [TRUE w897] -> w866
          frame False {
          }
          frame True {
            n439 = Two Button Dialog(message="The table has been modified.\nDo you want to continue?") -> (T button?=w897:bool)  [unwired: 2 in]
          }
        }
        n440 = case shown="True" w866 {
          tunnel: w867 -> [_ w873]
          frame False {
          }
          frame True {
            n441 = property on="Sub-Cycle List" class="LstBox (strict)"() -> ("Item Names"=w885:string[])  [unwired: 2 in, 2 out]
            n442 = Index Array(array=w885, index="Sub-Cycle List") -> (element=w872:string)
            n443 = Concatenate Strings(w873, w872) -> (w883:string)
            n444 = Search/Split String(string=w872, search string/char (-)=".") -> (substring before match=w870:string)  [unwired: 1 in, 2 out]
            n445 = local write "Sub-Cycle Name"(w870) -> ()
            n446 = String To Path(string=w883) -> (path=w882:path)
            n447 = call-poly <vilib>:"Read From Spreadsheet File.vi"("file path (dialog if empty)"=w882) -> ("first row"=w878:string[])  [unwired: 6 in, 4 out]
            n448 = Delete From Array(array=w878, length=1, index=0) -> (array with subset deleted=w875:string[])  [unwired: 1 out]
            n449 = Array Size(array=w875) -> (size(s)=w881:i32)
            n450 = Divide(x=w881, y=12) -> (x/y=w874:dbl)
            n451 = for {
              N: w874 -> [_]
              shift-right: [w891] -> _
              shift-left: w875 -> [w894]
              tunnel: [w890] -> w879 mode=indexing
              i -> [w889]
              n452 = Increment(x=w889) -> (x+1=w888:i32)
              n453 = Delete From Array(array=w894, length=12, index=0) -> (deleted portion=w886:string[], array with subset deleted=w891:string[])
              n454 = Number To Decimal String(number=w888) -> (decimal integer string=w887:string)  [unwired: 1 in]
              n455 = Build Array (concatenate)(w887, w886) -> (w890:string[])
            }
            n456 = local write "Sub-Cycle Pattern"(w879) -> ()
          }
        }
      }
      frame "delete subc" {
        n457 = Two Button Dialog(message="This operation will permanently delete this file!\nDo you want to continue?") -> (T button?=w901:bool)  [unwired: 2 in]
        n458 = case shown="True" w901 {
          tunnel: w902 -> [_ w907]
          frame False {
          }
          frame True {
            n459 = local read "Sub-Cycle List"() -> (w904:i32)
            n460 = property on="Sub-Cycle List" class="LstBox (strict)"() -> ("Item Names"=w905:string[])  [unwired: 2 in, 2 out]
            n461 = Index Array(array=w905, index=w904) -> (element=w909:string)
            n462 = Concatenate Strings(w907, w909) -> (w908:string)
            n463 = local write "Flag1"(FALSE) -> ()
            n464 = String To Path(string=w908) -> (path=w906:path)
            n465 = Delete(path (use dialog)=w906) -> ()  [unwired: 4 in, 3 out]
          }
        }
      }
      frame "clear table 2" {
        n466 = property on="Cycle Name" class="Str (strict)"("Value"="" ("Subcycle name")) -> ()  [unwired: 2 in, 2 out]
        n467 = local write "Flag 2"(FALSE) -> ()
        n468 = local write "Cycle Pattern"(string[][] [["", "", "", "", ""], ["", "", "", "", ""], ["", "", "", "", ""], ["", "", "", "", ""], ["", "", "", "", ""], ["", "", "", "", ""], ["", "", "", "", ""], ["", "", "", "", ""], ["", "", "", "", ""], ["", "", "", "", ""], ["", "", "", "", ""], ["", "", "", "", ""], ["", "", "", "", ""], ["", "", "", "", ""], ["", "", "", "", ""], ["", "", "", "", ""], ["", "", "", "", ""], ["", "", "", "", ""], ["", "", "", "", ""], ["", "", "", "", ""], ["", "", "", "", ""], ["", "", "", "", ""], ["", "", "", "", ""], ["", "", "", "", ""], ["", "", "", "", ""], ["", "", "", "", ""], ["", "", "", "", ""], ["", "", "", "", ""], ["", "", "", "", ""], ["", "", "", "", ""], ["", "", "", "", ""]]) -> ()
      }
      frame "update list 2" {
        n469 = String To Path(string=w915) -> (path=w916:path)
        n470 = List Folder(path=w916, pattern="*.eyec") -> (filenames=w914:string[])  [unwired: 2 in, 3 out]
        n471 = property on="Cycle List" class="LstBox (strict)"("Item Names"=w914) -> ()  [unwired: 2 in, 2 out]
      }
      frame "save cycle" {
        w917 = ".eyec" ("string")
        n472 = local read "Cycle Name"() -> (w918:T5)
        n473 = String To Path(string=w930) -> (path=w931:path)
        n474 = List Folder(path=w931, pattern="*.eyec" ("string")) -> (filenames=w929:string[])  [unwired: 2 in, 3 out]
        n475 = Equal?(x=w918, y="") -> (x = y?=w924:bool)
        n476 = Concatenate Strings(w918, w917) -> (w920:string)
        n477 = Search 1D Array(1D array=w929, element=w920) -> (index of element=w928:i32)  [unwired: 1 in]
        n478 = Concatenate Strings(w930, w918, w917) -> (w933:string)
        n479 = case shown="True" w924 {
          tunnel: [TRUE FALSE] -> w922
          frame False {
          }
          frame True {
            n480 = One Button Dialog(message="Insert file name!") -> ()  [unwired: 1 in, 1 out]
          }
        }
        n481 = String To Path(string=w933) -> (path=w932:path)
        n482 = Equal?(x=w928, y=-1) -> (x = y?=w926:bool)
        n483 = case shown="False" w926 {
          selector: w926 -> [_ w982]
          tunnel: [w980 w982] -> w923
          frame False {
            n484 = Two Button Dialog(message="A file with this name already exists!\nDo you want to overwrite?") -> (T button?=w980:bool)  [unwired: 2 in]
          }
          frame True {
          }
        }
        n485 = And(x=w923, y=w922) -> (x .and. y?=w921:bool)
        n486 = case shown="True" w921 {
          tunnel: w932 -> [_ w940]
          frame False {
          }
          frame True {
            n487 = local read "Cycle Pattern"() -> (w939:string[][])
            n488 = call "Table check.vi"("Input table"=w939) -> ("Incomplete?"=w937:bool, "Length"=w938:i32)  [unwired: 9 in]
            n489 = case shown="False" w937 {
              tunnel: w940 -> [w949 _]
              tunnel: w939 -> [w948 _]
              tunnel: w938 -> [w941 _]
              frame False {
                n490 = Number To Decimal String(number=w941) -> (decimal integer string=w944:string)  [unwired: 1 in]
                n491 = for {
                  N: w941 -> [_]
                  tunnel: w948 -> [w978]
                  shift-right: [w966] -> w945
                  shift-left: string[] [] -> [w976]
                  i -> [w977]
                  w957 = 12 ("length")
                  n492 = Index Array(array=w978, index (row)=w977) -> (element=w972:string[])  [unwired: 1 in]
                  n493 = Index Array(array=w972, index=3) -> (element=w962:string)
                  n494 = Index Array(array=w972, index=1) -> (element=w961:string)
                  n495 = Concatenate Strings("C:\\Setup Files\\Subcycles Folder\\", w961) -> (w973:string)
                  n496 = String To Path(string=w973) -> (path=w974:path)
                  n497 = call-poly <vilib>:"Read From Spreadsheet File.vi"("file path (dialog if empty)"=w974) -> ("first row"=w965:string[])  [unwired: 6 in, 4 out]
                  n498 = Delete From Array(array=w965, length=1, index=0) -> (array with subset deleted=w959:string[])  [unwired: 1 out]
                  n499 = String Length(string=w959) -> (length=w968:i32[])
                  n500 = Array Size(array=w968) -> (size(s)=w960:i32)
                  n501 = Divide(x=w960, y=w957) -> (x/y=w958:dbl)
                  n502 = Decrement(x=w958) -> (x-1=w950:dbl)
                  n503 = Multiply(x=w957, y=w950) -> (x*y=w956:dbl)
                  n504 = Number To Decimal String(number=w950) -> (decimal integer string=w967:string)  [unwired: 1 in]
                  n505 = Delete From Array(array=w959, length=12, index=w956) -> (deleted portion=w953:string[], array with subset deleted=w954:string[])
                  n506 = Index Array(array=w953, index=0) -> (element=w951:string)
                  n507 = Build Array (concatenate)(w961, w962, w967, w951, w954) -> (w971:string[])
                  n508 = Build Array (concatenate)(w976, w971) -> (w966:string[])
                }
                n509 = local write "Flag 2"(FALSE) -> ()
                n510 = Build Array (concatenate)("Cycle Data File for EYECAT - do not modify", w944, w945) -> (w946:string[])
                n511 = call-poly <vilib>:"Write To Spreadsheet File.vi"("1D data"=w946, "file path (dialog if empty)"=w949) -> ()  [unwired: 6 in, 1 out]
              }
              frame True {
                n512 = One Button Dialog(message="The table is incomplete!\nplease review and save again!") -> ()  [unwired: 1 in, 1 out]
              }
            }
          }
        }
      }
      frame "load cycle" {
        n513 = local read "Flag 2"() -> (w986:bool)
        n514 = case shown="True" w986 {
          tunnel: [w1025 w1027] -> w983
          tunnel: w985 -> [w1025 w1027]
          tunnel: [TRUE ("T button?") w1026] -> w984
          frame False {
          }
          frame True {
            n515 = Two Button Dialog(message="The table has been modified.\nDo you want to continue?") -> (T button?=w1026:bool)  [unwired: 2 in]
          }
        }
        n516 = case shown="True" w984 {
          tunnel: w983 -> [_ w989]
          frame False {
          }
          frame True {
            n517 = property on="Cycle List" class="LstBox (strict)"() -> ("Item Names"=w1005:string[])  [unwired: 2 in, 2 out]
            n518 = Index Array(array=w1005, index="Cycle List") -> (element=w991:string)
            n519 = Concatenate Strings(w989, w991) -> (w1004:string)
            n520 = Search/Split String(string=w991, search string/char (-)=".") -> (substring before match=w990:string)  [unwired: 1 in, 2 out]
            n521 = String To Path(string=w1004) -> (path=w1003:path)
            n522 = local write "Cycle Name"(w990) -> ()
            n523 = call-poly <vilib>:"Read From Spreadsheet File.vi"("file path (dialog if empty)"=w1003) -> ("first row"=w987:string[])  [unwired: 6 in, 4 out]
            n524 = Delete From Array(array=w987, length=2, index=0) -> (array with subset deleted=w988:string[])  [unwired: 1 out]
            n525 = Index Array(array=w987, index=1) -> (element=w1002:string)
            n526 = Decimal String To Number(string=w1002) -> (number=w1001:i32)  [unwired: 2 in, 1 out]
            n527 = for {
              N: w1001 -> [_]
              tunnel: w988 -> [w1023]
              tunnel: [w1018] -> w996 mode=indexing
              shift-right: [w1008] -> _
              shift-left: 0 ("x") -> [w1009]
              i -> [w1022]
              w1019 = ""
              n528 = Increment(x=w1009) -> (x+1=w1007:i32)
              n529 = Increment(x=w1007) -> (x+1=w1015:i32)
              n530 = Increment(x=w1022) -> (x+1=w1017:i32)
              n531 = Number To Decimal String(number=w1017) -> (decimal integer string=w1016:string)  [unwired: 1 in]
              n532 = Index Array(array=w1023, index #1=w1009, index #2=w1007, index #3=w1015) -> (element #1=w1021:string, element #2=w1020:string, element #3=w1014:string)
              n533 = Build Array(w1016, w1021, w1019, w1020, w1019) -> (w1018:string[])
              n534 = Decimal String To Number(string=w1014) -> (number=w1013:i32)  [unwired: 2 in, 1 out]
              n535 = Multiply(x=w1013, y=12 ("x")) -> (x*y=w1011:i32)
              n536 = Compound Arithmetic op=ADD(w1011, 4, w1009) -> (w1008:i32)
            }
            n537 = Insert Into Array(array=string[][] [["", "", "", "", ""], ["", "", "", "", ""], ["", "", "", "", ""], ["", "", "", "", ""], ["", "", "", "", ""], ["", "", "", "", ""], ["", "", "", "", ""], ["", "", "", "", ""], ["", "", "", "", ""], ["", "", "", "", ""], ["", "", "", "", ""], ["", "", "", "", ""], ["", "", "", "", ""], ["", "", "", "", ""], ["", "", "", "", ""], ["", "", "", "", ""], ["", "", "", "", ""], ["", "", "", "", ""], ["", "", "", "", ""], ["", "", "", "", ""], ["", "", "", "", ""], ["", "", "", "", ""], ["", "", "", "", ""], ["", "", "", "", ""], ["", "", "", "", ""], ["", "", "", "", ""], ["", "", "", "", ""], ["", "", "", "", ""], ["", "", "", "", ""], ["", "", "", "", ""], ["", "", "", "", ""]], index (row)=0, new element=w996) -> (w995:string[][])  [unwired: 1 in]
            n538 = local write "Cycle Pattern"(w995) -> ()
          }
        }
      }
      frame "delete cycle" {
        n539 = Two Button Dialog(message="This operation will permanently delete this file!\nDo you want to continue?") -> (T button?=w1031:bool)  [unwired: 2 in]
        n540 = case shown="True" w1031 {
          tunnel: w1030 -> [_ w1036]
          frame False {
          }
          frame True {
            n541 = local read "Cycle List"() -> (w1037:i32)
            n542 = property on="Cycle List" class="LstBox (strict)"() -> ("Item Names"=w1038:string[])  [unwired: 2 in, 2 out]
            n543 = Index Array(array=w1038, index=w1037) -> (element=w1035:string)
            n544 = Concatenate Strings(w1036, w1035) -> (w1034:string)
            n545 = String To Path(string=w1034) -> (path=w1033:path)
            n546 = Delete(path (use dialog)=w1033) -> ()  [unwired: 4 in, 3 out]
            n547 = local write "Flag 2"(FALSE) -> ()
          }
        }
      }
      frame "calc HC CO" {
        n548 = local read "Sub-Cycle Pattern"() -> (w1055:string[][])
        n549 = Index Array(array=w1055, index (col) #1=3 ("disabled index (col)"), index (col) #2=4 ("index (col)"), index (col) #3=11 ("index (col)")) -> (element #1=w1045:string[], element #2=w1052:string[], element #3=w1039:string[])  [unwired: 3 in]
        n550 = Array Size(array=w1045) -> (size(s)=w1043:i32)
        n551 = Search 1D Array(1D array=w1045, element="") -> (index of element=w1042:i32)  [unwired: 1 in]
        n552 = Equal?(x=w1042, y=-1) -> (x = y?=w1044:bool)
        n553 = Select(t=w1043, s=w1044, f=w1042) -> (s? t:f=w1041:i32)
        n554 = for {
          N: w1041 -> [_]
          tunnel: [w1066] -> w1049 mode=indexing
          tunnel: [w1065] -> w1048 mode=indexing
          tunnel: w1045 -> [w1064] mode=indexing
          tunnel: w1052 -> [w1063] mode=indexing
          tunnel: w1039 -> [w1062] mode=indexing
          w1061 = ""
          n555 = Not Equal?(x=w1064, y=w1061) -> (x != y?=w1060:bool)
          n556 = Not Equal?(x=w1063, y=w1061) -> (x != y?=w1059:bool)
          n557 = Not Equal?(x=w1062, y=w1061) -> (x != y?=w1058:bool)
          n558 = Compound Arithmetic op=AND(w1060, w1059, w1058) -> (w1057:bool)
          n559 = case shown="True" w1057 {
            tunnel: w1064 -> [_ w1095]
            tunnel: w1063 -> [_ w1094]
            tunnel: [w1067 w1091] -> w1065
            tunnel: [w1067 w1090] -> w1066
            tunnel: w1062 -> [_ w1068]
            frame False {
              w1067 = ""
            }
            frame True {
              # "O2Eq"
              n560 = Fract/Exp String To Number(string=w1068) -> (number=w1069:dbl)  [unwired: 3 in, 1 out]
              n561 = Fract/Exp String To Number(string=w1095) -> (number=w1076:dbl)  [unwired: 3 in, 1 out]
              n562 = Fract/Exp String To Number(string=w1094) -> (number=w1072:dbl)  [unwired: 3 in, 1 out]
              n563 = Decrement(x=w1076) -> (x-1=w1077:dbl)
              n564 = Divide(x=w1069, y=20000.0) -> (x/y=w1070:dbl)
              n565 = Multiply(x=4.76, y=w1076) -> (x*y=w1081:dbl)
              n566 = Multiply(x=w1077, y=100.0) -> (x*y=w1079:dbl)
              n567 = Add(x=w1072, y=w1070) -> (x+y=w1073:dbl)
              n568 = Add(x=0.33, y=w1081) -> (x+y=w1083:dbl)
              n569 = Divide(x=w1079, y=w1083) -> (x/y=w1084:dbl)
              n570 = Subtract(x=w1073, y=w1084) -> (x-y=w1086:dbl)
              n571 = Multiply(x=w1086, y=2.0) -> (x*y=w1074:dbl)
              n572 = Divide(x=w1086, y=5.0) -> (x/y=w1075:dbl)
              n573 = Number To Fractional String(number=w1075, width (-)=i16 6, precision (6)=i16 3) -> (F-format string=w1090:string)  [unwired: 1 in]
              n574 = Number To Fractional String(number=w1074, width (-)=i16 6, precision (6)=i16 2) -> (F-format string=w1091:string)  [unwired: 1 in]
            }
          }
        }
        n575 = Replace Array Subset(array=w1055, new element #1=w1049, index (col) #1=5 ("disabled index (col)"), new element #2=w1048, index (col) #2=6 ("disabled index (col)")) -> (w1053:string[][])  [unwired: 2 in]
        n576 = local write "Sub-Cycle Pattern"(w1053) -> ()
      }
      frame "Total time calc" {
        w1110 = i16 2 ("width (-)")
        w1117 = ":"
        n577 = local read "Cycle Pattern"() -> (w1124:string[][])
        n578 = Index Array(array=w1124, index (col)=4 ("disabled index (col)")) -> (element=w1097:string[])  [unwired: 1 in]
        n579 = Array Size(array=w1097) -> (size(s)=w1099:i32)
        n580 = Search 1D Array(1D array=w1097, element="") -> (index of element=w1098:i32)  [unwired: 1 in]
        n581 = Equal?(x=w1098, y=-1) -> (x = y?=w1100:bool)
        n582 = Select(t=w1099, s=w1100, f=w1098) -> (s? t:f=w1096:i32)
        n583 = for {
          N: w1096 -> [_]
          tunnel: w1097 -> [w1132] mode=indexing
          shift-right: [w1134] -> w1120
          shift-left: 0 -> [w1135]
          n584 = xnode "Match Regular Expression"("input string"=w1132, "regular expression"=":" ("search string/char (-)")) -> ("before match"=w1131:string, "after match"=w1128:string)  [unwired: 4 in, 3 out]
          n585 = Decimal String To Number(string=w1131) -> (number=w1130:i32)  [unwired: 2 in, 1 out]
          n586 = Decimal String To Number(string=w1128) -> (number=w1127:i32)  [unwired: 2 in, 1 out]
          n587 = Multiply(x=w1130, y=60) -> (x*y=w1126:i32)
          n588 = Add(x=w1126, y=w1127) -> (x+y=w1125:i32)
          n589 = Add(x=w1125, y=w1135) -> (x+y=w1134:i32)
        }
        n590 = local read "Total Number of Cycles"() -> (w1121:T1)
        n591 = Multiply(x=w1120, y=w1121) -> (x*y=w1116:T1)
        n592 = Quotient & Remainder(x=w1116, y=3600.0) -> (x-y*floor(x/y)=w1103:T1, floor(x/y)=w1113:T1)
        n593 = Quotient & Remainder(x=w1103, y=60.0) -> (x-y*floor(x/y)=w1111:T1, floor(x/y)=w1112:T1)
        n594 = Number To Decimal String(number=w1113) -> (decimal integer string=w1118:string)  [unwired: 1 in]
        n595 = Number To Decimal String(number=w1112, width (-)=w1110) -> (decimal integer string=w1114:string)
        n596 = Number To Decimal String(number=w1111, width (-)=w1110) -> (decimal integer string=w1109:string)
        n597 = Concatenate Strings(w1118, w1117, w1114, w1117, w1109) -> (w1108:string)
        n598 = call <vilib>:"Search and Replace Pattern.vi"("string"=w1108, "regular expression (\"\")"=" " ("replace string (\"\")"), "replace string (\"\")"="0" ("replace string (\"\")"), "replace all? (F)"=TRUE) -> ("result string"=→"Total Test Duration (hrs)":string)  [unwired: 1 in, 1 out]
      }
      frame "update Cycle pattern " {
        n599 = local read "Cycle Pattern"() -> (w1263:string[][])
        n600 = Index Array(array=w1263, index (col)=1 ("disabled index (col)")) -> (element=w1248:string[])  [unwired: 1 in]
        n601 = String To Path(string=w1265) -> (path=w1266:path)
        n602 = Array Size(array=w1248) -> (size(s)=w1251:i32)
        n603 = Search 1D Array(1D array=w1248, element="") -> (index of element=w1250:i32)  [unwired: 1 in]
        n604 = List Folder(path=w1266, pattern="*.eyes") -> (filenames=w1264:string[])  [unwired: 2 in, 3 out]
        n605 = Equal?(x=w1250, y=-1) -> (x = y?=w1252:bool)
        n606 = Select(t=w1251, s=w1252, f=w1250) -> (s? t:f=w1249:i32)
        n607 = for {
          N: w1249 -> [_]
          tunnel: w1263 -> [w1282] mode=indexing
          tunnel: w1265 -> [w1275]
          tunnel: [w1277] -> w1258 mode=indexing
          tunnel: [w1279] -> w1262 mode=indexing
          tunnel: [w1276] -> w1259 mode=indexing
          tunnel: w1264 -> [w1274]
          tunnel: [w1269] -> w1255 mode=indexing
          n608 = Index Array(array=w1282, index #1=1 ("index"), index #2=3 ("index")) -> (element #1=w1273:string, element #2=w1278:string)
          n609 = Search 1D Array(1D array=w1274, element=w1273) -> (index of element=w1272:i32)  [unwired: 1 in]
          n610 = Not Equal?(x=w1272, y=-1) -> (x != y?=w1270:bool)
          n611 = case shown="True" w1270 {
            tunnel: [w1286 w1300] -> w1279
            tunnel: w1278 -> [_ w1296]
            tunnel: [w1286 w1294] -> w1277
            tunnel: [w1286 w1293] -> w1276
            tunnel: w1275 -> [_ w1292]
            tunnel: w1273 -> [w1285 w1291]
            tunnel: [w1284 w1291] -> w1269
            frame False {
              w1286 = "N/A" ("String")
              n612 = Concatenate Strings(w1285, " - File NOT AVAILABLE !!!" ("string")) -> (w1284:string)
            }
            frame True {
              w1304 = i16 2 ("width (-)")
              n613 = Concatenate Strings(w1292, w1291) -> (w1322:string)
              n614 = String To Path(string=w1322) -> (path=w1321:path)
              n615 = call <vilib>:"Search and Replace Pattern.vi"("string"=w1296, "regular expression (\"\")"="[a-x ]" ("format string"), "replace string (\"\")"="", "replace all? (F)"=TRUE) -> ("result string"=w1293:string)  [unwired: 1 in, 1 out]
              n616 = call-poly <vilib>:"Read From Spreadsheet File.vi"("file path (dialog if empty)"=w1321) -> ("first row"=w1290:string[])  [unwired: 6 in, 4 out]
              n617 = Delete From Array(array=w1290, length=1, index=0) -> (array with subset deleted=w1289:string[])  [unwired: 1 out]
              n618 = Array Size(array=w1289) -> (size(s)=w1320:i32)
              n619 = Equal?(x=w1293, y="") -> (x = y?=w1308:bool)
              n620 = Subtract(x=w1320, y=12) -> (x-y=w1318:i32)
              n621 = Select(t="0", s=w1308, f=w1293) -> (s? t:f=w1307:string)
              n622 = Index Array(array=w1289, index=w1318) -> (element=w1294:string)
              n623 = Decimal String To Number(string=w1307) -> (number=w1317:i32)  [unwired: 2 in, 1 out]
              n624 = Decimal String To Number(string=w1294) -> (number=w1316:i32)  [unwired: 2 in, 1 out]
              n625 = Multiply(x=w1317, y=w1316) -> (x*y=w1315:i32)
              n626 = Quotient & Remainder(x=w1315, y=60) -> (x-y*floor(x/y)=w1313:i32, floor(x/y)=w1312:i32)
              n627 = Number To Decimal String(number=w1313, width (-)=w1304) -> (decimal integer string=w1310:string)
              n628 = Number To Decimal String(number=w1312, width (-)=w1304) -> (decimal integer string=w1309:string)
              n629 = Concatenate Strings(w1309, ":", w1310) -> (w1303:string)
              n630 = call <vilib>:"Search and Replace Pattern.vi"("string"=w1303, "regular expression (\"\")"=" " ("replace string (\"\")"), "replace string (\"\")"="0" ("replace string (\"\")"), "replace all? (F)"=TRUE) -> ("result string"=w1300:string)  [unwired: 1 in, 1 out]
            }
          }
        }
        n631 = Replace Array Subset(array=w1263, new element #1=w1255, index (col) #1=1 ("disabled index (col)"), new element #2=w1258, index (col) #2=2 ("disabled index (col)"), new element #3=w1259, index (col) #3=3 ("disabled index (col)"), new element #4=w1262, index (col) #4=4 ("disabled index (col)")) -> (w1267:string[][])  [unwired: 4 in]
        n632 = local write "Cycle Pattern"(w1267) -> ()
      }
      frame "load cycle name" {
        n633 = property on="Cycle Pattern" class="Tbl (strict)"() -> ("EditPos"=w1328:T3)  [unwired: 2 in, 2 out]
        n634 = Unbundle By Name(w1328) -> ("Row"=w1326:i32, "Column"=w1325:i32)
        n635 = local read "Cycle Pattern"() -> (w1324:string[][])
        n636 = call "SubCycles list.vi"() -> ("Subcycle name"=w1327:string)  [unwired: 10 in, 1 out]
        n637 = Replace Array Subset(array=w1324, new element=w1327, index (row)=w1326, index (col)=w1325) -> (w1323:string[][])
        n638 = local write "Cycle Pattern"(w1323) -> ()
      }
      frame "load test array" {
        n639 = local read "Total Test Duration (hrs)"() -> (w1336:T8)
        n640 = local read "Cycle Name"() -> (w1332:T5)
        n641 = Equal?(x=w1332, y="") -> (x = y?=w1331:bool)
        n642 = Not Equal?(x=w1336, y="0:00:00") -> (x != y?=w1330:bool)
        n643 = Or(x=w1330, y=w1331) -> (x .or. y?=w1329:bool)
        n644 = case shown="True" w1329 {
          selector: w1329 -> [w1337 _]
          tunnel: [FALSE TRUE] -> w1334
          frame False {
            n645 = case shown="False" w1337 {
              frame False {
                n646 = One Button Dialog(message="Incomplete Data!\nReview the cycle pattern!") -> ()  [unwired: 1 in, 1 out]
              }
              frame True {
              }
            }
          }
          frame True {
            w1343 = 0.0 ("default (0 I32)")
            n647 = local read "Cycle Name"() -> (w1358:T5)
            n648 = Concatenate Strings("C:\\Setup Files\\Cycles Folder\\", w1358, ".eyec" ("string")) -> (w1356:string)
            n649 = String To Path(string=w1356) -> (path=w1357:path)
            n650 = local read "Total Number of Cycles"() -> (w1354:T1)
            n651 = call-poly <vilib>:"Read From Spreadsheet File.vi"("file path (dialog if empty)"=w1357) -> ("first row"=w1340:string[])  [unwired: 6 in, 4 out]
            n652 = call "Remove names.vi"("Array in"=w1340) -> ("Array out"=w1349:string[])  [unwired: 10 in]
            n653 = Index Array(array=w1340, index #1=14 ("index"), index #2=15 ("index")) -> (element #1=w1345:string, element #2=w1341:string)
            n654 = Number To Decimal String(number="Ageing Gas") -> (decimal integer string=w1353:string)  [unwired: 1 in]
            n655 = Number To Decimal String(number=w1354) -> (decimal integer string=w1352:string)  [unwired: 1 in]
            n656 = Decimal String To Number(string=w1341, default (0L)=w1343) -> (number=w1342:dbl)  [unwired: 1 in, 1 out]
            n657 = Decimal String To Number(string=w1345, default (0L)=w1343) -> (number=w1344:dbl)  [unwired: 1 in, 1 out]
            n658 = property on="Inlet temp Age" class="DigNum (strict)"("Value"=w1344) -> ()  [unwired: 2 in, 2 out]
            n659 = property on="Flow rate Age" class="DigNum (strict)"("Value"=w1342) -> ()  [unwired: 2 in, 2 out]
            n660 = Build Array (concatenate)(w1353, w1352, w1349) -> (w1348:string[])
            n661 = shared-variable "My Computer\\Library 1.lvlib\\Ageing Variables"(w1348) -> ()  [unwired: 1 in, 1 out]
          }
        }
        "Test Compiled" <- w1334
      }
      frame "convert to num" {
        n662 = local read "EditPos Subc"() -> (w1363:T3)
        n663 = Unbundle By Name(w1363) -> ("Row"=w1364:i32, "Column"=w1361:i32)
        n664 = Equal?(x=w1361, y=7) -> (x = y?=w1360:bool)
        n665 = case shown="False" w1360 {
          tunnel: w1364 -> [_ w1369]
          tunnel: w1361 -> [_ w1367]
          tunnel: w1363 -> [_ _]
          frame True {
          }
          frame False {
            n666 = local read "Sub-Cycle Pattern"() -> (w1366:string[][])
            n667 = call "Conv to num.vi"("Column"=w1367, "Row"=w1369, "Array"=w1366) -> ("result string"=w1368:string)  [unwired: 8 in]
            n668 = Replace Array Subset(array=w1366, new element=w1368, index (row)=w1369, index (col)=w1367) -> (w1365:string[][])
            n669 = local write "Sub-Cycle Pattern"(w1365) -> ()
          }
        }
      }
      frame "check scycle name" {
        n670 = local read "Sub-Cycle Name"() -> (w1370:T5)
        n671 = call <vilib>:"Search and Replace Pattern.vi"("string"=w1370, "regular expression (\"\")"="[^0-9a-zA-Z ]" ("format string"), "replace string (\"\")"="", "replace all? (F)"=TRUE) -> ("result string"=w1376:string)  [unwired: 1 in, 1 out]
        n672 = Not Equal?(x=w1376, y=w1370) -> (x != y?=w1375:bool)
        n673 = case shown="False" w1375 {
          tunnel: w1376 -> [w1377 w1378]
          tunnel: [w1377 w1378] -> w1371
          frame False {
          }
          frame True {
            n674 = One Button Dialog(message="Unsuitable character for the file name!") -> ()  [unwired: 1 in, 1 out]
          }
        }
        n675 = local write "Sub-Cycle Name"(w1371) -> ()
      }
      frame "check cycle name" {
        n676 = local read "Cycle Name"() -> (w1380:T5)
        n677 = call <vilib>:"Search and Replace Pattern.vi"("string"=w1380, "regular expression (\"\")"="[^0-9a-zA-Z ]" ("format string"), "replace string (\"\")"="", "replace all? (F)"=TRUE) -> ("result string"=w1386:string)  [unwired: 1 in, 1 out]
        n678 = Not Equal?(x=w1386, y=w1380) -> (x != y?=w1385:bool)
        n679 = case shown="False" w1385 {
          tunnel: w1386 -> [w1387 w1388]
          tunnel: [w1387 w1388] -> w1381
          frame False {
          }
          frame True {
            n680 = One Button Dialog(message="Unsuitable character for the file name!") -> ()  [unwired: 1 in, 1 out]
          }
        }
        n681 = local write "Cycle Name"(w1381) -> ()
      }
      frame "Multigas connect" {
        # "add here logic to verify the user requirements and the machine state\n0 - not connected\n1 - MKS1 & Ext An Up\n2 - MKS2 & Ext An Dn\n3 - MKS 1 & 2  & Ext An Up & Dn"
        n682 = flat-sequence {
          frame #0 {
            "Connected?" <- TRUE
          }
        }
      }
      frame "Multigas disconnect" {
      }
    }
    n683 = local read "stop 2"() -> (w766:bool)
  }
  n684 = node-c288(w2) -> ()  [unwired: 1 out]
  n685 = local write "stop 2"(w12) -> ()
  n686 = node-c288(w9) -> ()  [unwired: 1 out]
  "Table" <- string[][] [] ("Table")
